vi "UHR-Fleezers Control (fpga) - Leonardo 04-2018 V5.2.vi"() -> ()   [LabVIEW 2013]
doc: "UHR-Fleezers Instrument Control Code (fpga)"
uses:
  <vilib>/Platform/TimedLoop/XDataNode/timing_clust.ctl
  <vilib>/Platform/TimedLoop/XDataNode/nitl_modes.ctl
  <vilib>/Platform/TimedLoop/XDataNode/wakeup.ctl
  <vilib>/rvi/eio/common/nirviEmuTemplateMethod_errors.vi
  <vilib>/rvi/Emulation/niFpgaSctlEmulationGetInTimedLoop.vi
  <vilib>/rvi/Emulation/niFpgaEmulationReportErrorSimple.vi
  <vilib>/rvi/Emulation/niFpgaGetClockAttributes.vi
  <vilib>/rvi/Emulation/niFpgaCriticalErrorInLSC.vi
  <vilib>/rvi/FIFO/Fifo_Resource/nirvififoEmulationReadFpgaImpl.vi
  <vilib>/rvi/DataTransferAndStorage/Container/Common/niFpgaContainerGetUniqueNameForEmu.vi
  <vilib>/rvi/DataTransferAndStorage/Container/Common/niFpgaContainerExecOnDevCompGetState.vi
  <vilib>/rvi/interface/RandomDataEmulation/nirviRandomDataFPGAFIFO.vi
  <vilib>/rvi/interface/RandomDataEmulation/niFpgaRandomDataHandleErrors.vi
  <vilib>/rvi/eio/common/nirviEmuReportErrorAndStop.vi
  <vilib>/rvi/Emulation/niFpgaProcessEmulError.vi
  <vilib>/rvi/FIFO/Fifo_Resource/nirvififoEmulationWriteFpgaImpl.vi
  <vilib>/Platform/TimedLoop/XDataNode/XDataNode.xnode
  <vilib>/eio/EIOMethodNode/EIOMethodNode.xnode
  <vilib>/eio/EIONode/EIONode.xnode
  <vilib>/rvi/DataTransferAndStorage/Container/XNode/niFpgaContainer.xnode
  <vilib>/rvi/FIFO/Fifo_Resource/nirvififoEmulationRead.vi
  <vilib>/rvi/FIFO/Fifo_Resource/niFpgaFifoEmulationRefIn.vi
  <vilib>/rvi/interface/RandomDataEmulation/nirviRandomDataFpgaReadWriteTemplate.vi
  <vilib>/rvi/FIFO/Fifo_Resource/nirvififoEmulationWrite.vi
  <vilib>/addons/control/pid/fpga.llb/XNode/niFpgaPID.xnode
  <vilib>/Platform/TimedLoop/XDataNode/XDNodeRunTimeDep.lvlib
  <vilib>/rvi/Memory/Memory_Emulation/niFpgaMemoryEmulationRefIn.vi
panel:
  in  "Symmetric FB/Raster":bool
  in  "Tab Control 2":T1(tab)
  out "BD1 amplitude 1 out":u16
  out "BD1 amplitude 2 out":u16
  in  "FB output range":cluster{"output low":i16, "output high":i16}={"output low"=0, "output high"=3000}
  in  "FB Gains":T2={"proportional gain (Kc)"=10, "integral gain (Kc*Ts/Ti)"=5, "derivative gain (Kc*Td/Ts)"=0}
  in  "RF synth green feedback max":i16=4000
  in  "RD":bool=TRUE
  in  "Swap F1 and F2":bool
  in  "Scan BD":bool
  in  "Start scan":bool
  in  "OSK Bd 1":bool
  in  "Reset Bd 1":bool
  in  "PMODE":bool=TRUE
  in  "Number Interlace Cycles":u8=2 min=1 max=3
  in  "Interlace Off Parameters":u8=1 min=1 max=3
  in  "Interlace ON/OFF":bool
  out "DIO Relative phase":i16
  in  "Phase count adjustment (DIO)":i16
  in  "+ phase (DIO)":bool
  out "DIO Late Counter":u8
  in  "DIO count 1 (ticks)":u16=400
  in  "DIO count 2 (ticks)":u16=400
  in  "DIO count 3 (ticks)":u16=400
  out "AI2 Y Sum Set 2":i16
  out "AI2 Y Sum Set 1":i16
  in  "FB Setpoint Set 1":i16 min=0 step=1
  in  "FB Reset Set 1":bool
  in  "FB On/Off Set 1":bool
  in  "FB Reset Set 2":bool
  in  "FB On/Off Set 2":bool
  in  "FB Setpoint Set 2":i16 min=0 step=1
  in  "Amp switch delay":u8=5
  in  "RF synth bd controls green":bool
  in  "Phase Trap 2":fxp<+,14,14>
  in  "Phase Trap 1":fxp<+,14,14>
  in  "Phase offset method":u8
  in  "BD 2 Amplitude 1":u16
  in  "BD 1 Amplitude 1":u16
  in  "BD 2 Frequency 1":u64
  in  "BD 1 Frequency 1":u64
  in  "BD 2 Amplitude 2":u16
  in  "BD 1 Amplitude 2":u16
  in  "BD 2 Frequency 2":u64
  in  "BD 1 Frequency 2":u64
  in  "BD 2 Amplitude 3":u16
  in  "BD 1 Amplitude 3":u16
  in  "BD 2 Frequency 3":u64
  in  "BD 1 Frequency 3":u64
  in  "BD 2 Delay (Ticks)":u8 caption="Count(Ticks)"
  in  "Next trap write delay (ticks)":u8 caption="Count(Ticks)"
  out "Random phase generated":fxp<+,14,14>
  in  "RF phase reset before cycles":bool
  in  "Trap 1 osc enable":bool
  in  "N trap osc periods":i16
  in  "Trap osc period (pts)":i16
  in  "Osc traps":bool
  in  "Initiate trap osc":bool
  in  "Ready Write":bool
  in  "Data":i64
  in  "Address 2":u32
  in  "Osc trap cont.":bool
  in  "Trap 2 osc enable":bool
  out "green FB running":bool
  in  "APD 2 AO scale factor":i16=1
  in  "BD 1 Delay (ticks)":u8
  in  "Tab Control":T3(tab)=enum."MCL trap control"
  in  "Set 3":bool
  in  "Set 2":bool=TRUE
  in  "Set 1":bool=TRUE
  in  "Trap Pos to FIFO":bool
  in  "N of AI1 Int Acq Sets":i16=2 min=1 max=3 step=1
  out "AI Late Counter":u8
  in  "ai count":u16=400
  in  "+ phase":bool
  in  "Phase count adjustment":i16
  out "Relative phase":i16
  in  "AI to FIFO":bool
  out "BD1 Frequency Out 1":u64
  out "BD1 Frequency Out 2":u64
  out "Trap Pos FIFO Timeout":u16
  out "Trap AI FIFO Timeout":u16
  in  "Trap FIFO Set Timeout":i32
  in  "Scan freq.  increment":i64
  in  "Scan steps":u64
  in  "Number of scans":u16
  in  "Cycles per step":u64
  in  "Raster setpoint":fxp<+/-,16,1>
  in  "Raster to target force":bool
  out "Actual Scan freq":u64
  in  "Cont. Scan":bool
  out "Scan I":u64
  in  "Abort scan":bool
  out "Scanning":bool
  in  "FB Min frequency":u64
  in  "FB Max Frequency":u64
  in  "Dynamic Force FB (Ronen)":bool
  in  "Trap pos. FB Range":T4={"FB2 output low"=-1.0, "FB2 output high"=0.999969482421875}
  in  "Trap Pos. FB Gains":T5={"proportional gain (Kc)"=0.999969482421875, "integral gain (Kc*Ts/Ti)"=0.999969482421875, "derivative gain (Kc*Td/Ts)"=0.0}
  in  "B factor":fxp<+/-,32,16>
  in  "Negate Diff?":bool
  in  "Diff FB Measurement?":bool
  in  "FB Trig Integrate":u32=1
  out "TTrig?":bool
  in  "TTrig Negate Pos":bool=TRUE
  out "Trap Pos FB Int Signal":fxp<+/-,24,9> format="%.18g"
  out "Trap Pos FB Int-Norm Signal":fxp<+/-,16,1> format="%.16g"
  in  "FPGA TTrig Thresh":i64
  in  "FPGA Trap Trig":bool
  out "Trap Pos FB Action":i64
  in  "Trap Pos. FB Offset Factor":i64
  in  "Trap Pos. FB Mult Factor":i64=2
  in  "Trap Pos. FB Reset":bool
  in  "Trap Pos FB Monitor T1 or T2":bool
  in  "AI1 X Scale":u16
  in  "Trap Pos FB Int Count":u16=100
  in  "Trap Pos FB Negate Action":bool
  out "AI1 X Set 2":fxp<+/-,16,1>
  out "AI1 X Set 1":fxp<+/-,16,1>
  in  "Trap Pos. FB SP":fxp<+/-,16,1>
  in  "Force feedback":bool
  out "TTrig Sig":i64
  out "TTrig Fin Thresh":i64
  in  "1D or 2D Scan?":bool
  in  "Abort scan (MCL)":bool
  in  "MCL Scan Axis":bool
  in  "Cont. Scan (MCL)":bool
  out "Scan I (MCL)":u64
  in  "Number of scans (MCL)":u16
  out "Scanning MCL":bool
  in  "Scan steps (MCL)":u64
  in  "Cycles per step (MCL)":u64
  in  "Scan freq.  increment (MCL)":i16
  in  "Start scan (MCL)":bool
  in  "AO2 (X)":i16
  in  "AO1 (Y)":i16
  out "MCL Late Counter":u8
  in  "MCL count":u32=800
  out "MCL Relative Phase":i16
  in  "Phase count adjustment (MCL)":i16
  in  "+ phase (MCL)":bool
  in  "Lifetime events to read blue":u16=100
  in  "Lifetime read blue fifo":bool
  out "lifetime events in fifo":u16
  out "APD2 int gate":bool
  in  "APD Gate Operating Mode":u8 max=2 step=1
  in  "Invert APD Gate":bool
  in  "APD Gate OFF Count":u16=100
  in  "APD Gate ON Count":u16=300
  out "APD 1 Gate Late Counter":u8
  out "APD 1 Gate Relative Phase":i16
  in  "Phase count adjustment (APD 1 Gate)":i16
  in  "+ phase (APD 1 Gate)":bool
  out "APD 2 Counts 0":u32
  out "APD 2 Counts 1":u32
  out "APD 1 Counts 0":u32
  out "APD 1 Counts 1":u32
  in  "Phase count adjustment (APD 2 Gate)":i16
  out "APD 2 Gate Late Counter":u8
  out "APD 2 Gate Relative Phase":i16
  in  "+ phase (APD 2 Gate)":bool
  out "APD 3 Counts 0":u32
  out "APD 3 Counts 1":u32
  out "APD 3 Gate Late Counter":u8
  in  "Phase count adjustment (APD 3 Gate)":i16
  out "APD 3 Gate Relative Phase":i16
  in  "+ phase (APD 3 Gate)":bool
  out "APD1 int gate":bool
  out "APD3 int gate":bool
  in  "Lifetime timeout APD1":u16=200
  in  "APD to FIFO":bool
  in  "APD Acq Rate Count":u32=20000000
  out "APD Acq Late Counter":u16
  out "APD Acq Relative Phase":i16
  in  "+ phase (APD Acq)":bool
  in  "Phase Count Adjustment (APD Acq)":i16
  in  "APD 1 AO scale factor":i16=1
  out "APD2 out state":bool
  out "APD1 out state":bool
  out "APD Acq Late?":bool
  in  "Number of OFF cycles":i16
  in  "Green long-scale interlacing":bool
  in  "D3 2":i16
  in  "I3 2":i16=5
  in  "P3 2":i16=10
  in  "Green FB Setpoint 2":i16=250 min=0 step=1
  in  "Green FB Reset 2":bool
  in  "Green Filter Flipper":bool
  in  "Green interlace OFF count":u16=100
  out "GI Relative phase":i16
  in  "Phase count adjustment (GI)":i16
  in  "+ phase (GI)":bool
  in  "Green interlace ON count":u16=300
  out "GI Late Counter":u8
  in  "Invert GI":bool
  in  "Operating Mode":u8 max=2 step=1
  in  "Current Out":u16=30000
  in  "Green int current ON count adj":u32=150
  in  "Green interlace OFF count 2":u32=900
  in  "Green interlace ON count 2":u32=300
  out "GI Late Counter 2":u16
  in  "Green FB Count":u32=1200
  in  "Phase count adjustment (GI) 2":i16=20
  in  "Green FB Setpoint":i16=250 min=0 step=1
  in  "Invert GI 2":bool
  out "GI Relative phase 2":i16
  in  "+ phase (GI) 2":bool
  in  "Phase count adjustment (Green FB)":i16=10
  out "Green Late Counter":u16
  out "Green FB Relative Phase":i16
  in  "+ phase (Green FB)":bool
  out "Green FB Signals":T6
  out "Green FB Sum":i16
  in  "Green FB Gains":T2={"proportional gain (Kc)"=10, "integral gain (Kc*Ts/Ti)"=5, "derivative gain (Kc*Td/Ts)"=0}
  in  "Green FB On/Off":bool
  in  "Green FB Reset":bool
  out "Green FB Late?":bool
  out "GI Late?":bool
  in  "Operating Mode 2":u8=2 max=2 step=1
  in  "Chassis2/Mod4/AO1":u16
  in  "Number of ON cycles":i16
  in  "+ phase (RI)":bool
  out "RI Relative phase":i16
  out "RI Late Counter":u8
  in  "Red interlace ON count":u16=300
  in  "Red interlace OFF count":u16=100
  in  "Invert RI":bool
  in  "Red Laser Operating Mode":u8 max=2 step=1
  in  "Phase count adjustment (RI)":i16
  in  "Phase count adjustment (BI D)":i16
  in  "Blue Laser Operating Mode (D)":u8 max=2 step=1
  in  "Invert BI (D)":bool
  in  "Blue interlace OFF count (D)":u16=100
  in  "Blue interlace ON count (D)":u16=300
  out "Blue Late Counter (D)":u8
  out "BI Relative phase (D)":i16
  in  "+ phase (BI D)":bool
  in  "Lifetime to FIFO":bool
  out "lifetime (ticks)":u16
  # "Raster Scan AOD"
  # "1 (X)"
  # "2 (Y)"
  # "IR Intensity Feedback (RF BD 1)"
  # "FB Gains Set 1"
  # "FB output range 1"
  # "IR Intensity Feedback (RF BD 2) -\nonly when using BD 2 for green laser AOM (not trap Y)"
  # "Keep below 4096 (12 bits) to stay within range of RF board. Going over doesn't saturate, it truncates higher bits."
  # "RF phase offset control"
  # "Methods are:\n0 - Default, do nothing at all (no phase offset writes)\n1 - Manual phase adjustment\n2 - Cycle the phase adjustment using the input phase numbers as increment values for each cycle"
  # "False is usual, True is external loop method"
  # "Parameters if using the external RF switching loop"
  # "Parameters if using the usual internal RF switching method"
  # "FB Triggering Excitation Laser"
  # "Trap Pos. FB Gains"
  # "Trap Pos. FB Range"
  # "AO1 (Y)"
  # "2D"
  # "Trap 3"
  # "1D"
  # "AO2 (X)"
  # "Fl Laser"
  # "APD AO for aligning"
  # "Detection Loop"
  # "Green fluorescent laser digital gate interlacing loop"
  # "0 Forced ON\n1 Forced OFF\n2 Interlacing"
  # "ALEX settings:"
  # "Controls for usual IA ME controls green AOM"
  # "Controls for RF synth board controls green AOM"
  # "Green FB Gains"
  # "Red fluorescent laser digital gate interlacing loop"
  # "Detection Loop"
  # "0 Forced ON\n1 Forced OFF\n2 Interlacing"
  # "Analog/FB Control Loop\n(Disabled)"
  # "Digital Control Loop"
  # "Blue laser intensity reading"
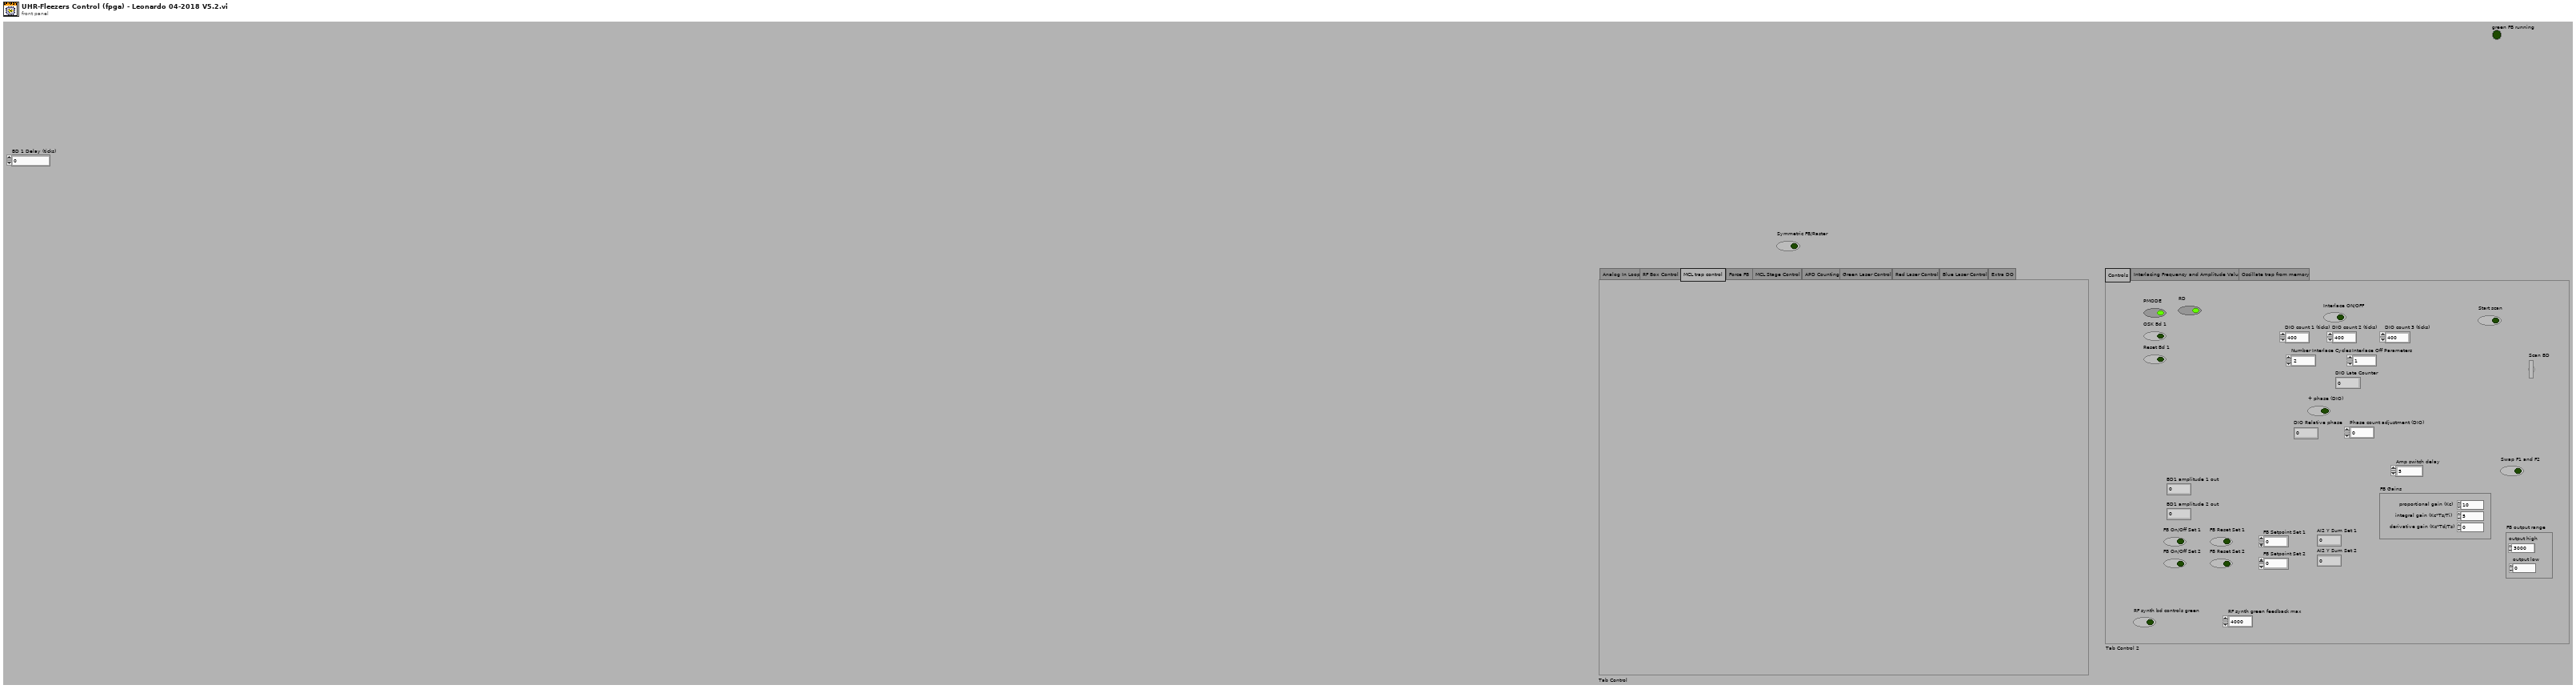
[diagram p1: front panel]
types:
  T1 = enum32{"Controls", "Interlacing Frequency and Amplitude Values", "Oscillate trap from memory"}
  T2 = cluster{"proportional gain (Kc)":i16, "integral gain (Kc*Ts/Ti)":i16, "derivative gain (Kc*Td/Ts)":i16}
  T3 = enum32{"Analog In Loop", "RF Box Control", "MCL trap control", "Force FB", "MCL Stage Control", "APD Counting", "Green Laser Control", "Red Laser Control", "Blue Laser Control", "Extra DO"}
  T4 = cluster{"FB2 output low":fxp<+/-,16,1>, "FB2 output high":fxp<+/-,16,1>}
  T5 = cluster{"proportional gain (Kc)":fxp<+/-,16,1>, "integral gain (Kc*Ts/Ti)":fxp<+/-,16,1>, "derivative gain (Kc*Td/Ts)":fxp<+/-,16,1>}
  T6 = cluster{"Green FB Ch 0":i16, "Green FB Ch 1":i16, "Green FB Ch 2":i16}
  T7 = typedef "XDNodeRunTimeDep.lvlib/timing_clust.ctl" = cluster{"Expected End [f-1]":u64, "Actual End [f-1]":u64, "Finished Late? [f-1]":bool, "Expected End [i-1]":u64, "Actual End [i-1]":u64, "Finished Late? [i-1]":bool, "Expected Start [i]":u64, "Actual Start [i]":u64, "Expected Start [f]":u64, "Actual Start [f]":u64, "Source Name":string, "Structure Name":string, "Period":i64, "Deadline":i64, "Offset":i64, "Start":i64, "Priority":i32, "Timeout":i32, "Mode":T8, "Wakeup Reason":T9, "Error":errorcluster, "Source Type":string, "Secondary Source Type":string, "Global End Time":u64, "Global Start Time":u64, "Frame Duration":u64, "Iteration Duration":u64, "Assigned CPU":i32, "I/O Scan Engine Mode":u32}
  T8 = typedef "XDNodeRunTimeDep.lvlib/nitl_modes.ctl" = enum32{"No Change", "Process missed periods, maintain original phase", "Discard missed periods, maintain original phase", "Process missed periods, ignore original phase", "Discard missed periods, ignore original phase"}
  T9 = typedef "XDNodeRunTimeDep.lvlib/wakeup.ctl" = enum32{"Normal", "Aborted", "Asynchronous wakeup", "Timing source error", "Timed loop error", "Timeout"}
  T10 = cluster{"Chassis2/Mod2/AI0":i16, "Chassis2/Mod2/AI1":i16, "Chassis2/Mod2/AI2":i16}
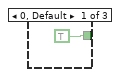
[diagram p2: hidden frame]
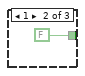
[diagram p3: hidden frame]
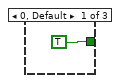
[diagram p6: hidden frame]
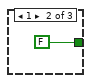
[diagram p7: hidden frame]
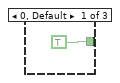
[diagram p11: hidden frame]
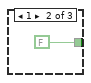
[diagram p12: hidden frame]
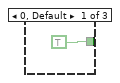
[diagram p13: hidden frame]
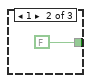
[diagram p14: hidden frame]
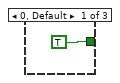
[diagram p18: hidden frame]
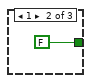
[diagram p19: hidden frame]
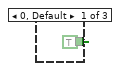
[diagram p20: hidden frame]
diagram:
  w4 = FALSE
  w5 = FALSE
  # "BD2 amp"
  # "BD1 amp"
  # "BD2 amp"
  # "BD1 amp"
  # "timing array current index"
  # "timing array"
  # "timing counter (phase adjusted here)"
  # "late counter"
  n1 = while {
    stop <- FALSE stop-if-true
    n2 = xnode "FPGA I/O Node"("Connector0/DIO3"="Green Filter Flipper", "Chassis2/Mod1/AO1"="Chassis2/Mod4/AO1") -> ()  [unwired: 2 in, 2 out]
    n3 = call "Loop Timer11"("Count(Ticks)"=u32 40000 ("Extra DO Counts")) -> ()  [unwired: 1 out]
  }
  n4 = disable-structure shown="Disabled" {
    frame Disabled {
      w19 = i16 2 items=["UnSet Ready", "ReadWrite", "Wait Ready"]
      n5 = while "Handshake memory transfer for trap oscillation sin wave data" {
        shift-right: [w21] -> _
        shift-left: w19 -> [w22]
        stop <- FALSE stop-if-true
        # "Write"
        n6 = case shown="1" w22 {
          tunnel: [w25 w30 w31] -> w21
          frame 3, Default {
            w23 = i16 2 items=["UnSet Ready", "ReadWrite", "Wait Ready"]
            w24 = i16 1 items=["UnSet Ready", "ReadWrite", "Wait Ready"]
            n7 = Select(t=w24, s="Ready Write", f=w23) -> (s? t:f=w25:i16)
          }
          frame 1 {
            w30 = i16 0 items=["UnSet Ready", "ReadWrite", "Wait Ready"]
            n8 = xnode ("Memory Write")("Address"="Address 2", "Data"="Data", "Memory In"=refnum<k21> "Trap osc memory") -> ()  [unwired: 1 out]
          }
          frame 0 {
            w31 = i16 2 items=["UnSet Ready", "ReadWrite", "Wait Ready"]
            n9 = local write "Ready Write"(FALSE ("Ready Read")) -> ()
          }
        }
      }
    }
    frame Enabled {
    }
  }
  n10 = flat-sequence "FPGA initialization to do before running any of the loops" {
    tunnel: [u16 0 ("DIO count 3 (ticks)")] -> w3
    tunnel: [w40] -> _
    frame #0 {
      # "UDCLK out enable and set low"
      # "WR"
      # "BD 2"
      # "BD 1"
      # "With the RF synth board initialization now done in a separate fpga vi, now when this vi is started, board is already configured and is ready for interlacing. Just need to set WR high and enabled UDCLK as write and set to low.\nbefore setting data and address bits."
      # "Start up expansion chassis early\nto avoid delays later"
      # "Set data and address values to something safe (a correct setting) so any initial WR and udclk flipping doesn't have a chance to mess anything up. Safe would be setting an unused data entry:"
      n11 = xnode "FPGA I/O Method Node"("Enable"=TRUE) -> ("FPGA I/O Out"=w34:refnum<k21>)  [unwired: 1 in]
      n12 = xnode "FPGA I/O Method Node"("Enable"=TRUE) -> ("FPGA I/O Out"=w37:refnum<k21>)  [unwired: 1 in]
      n13 = xnode "FPGA I/O Node"("Chassis2/Mod1/AO0"=u16 0 ("Chassis2/Mod4/AO0")) -> ("Chassis2/Mod2/AI0"=w40:i16)  [unwired: 2 in, 2 out]
      n14 = xnode "FPGA I/O Node"("Connector1/DIO15"=TRUE) -> ()  [unwired: 1 in, 1 out]
      n15 = xnode "FPGA I/O Node"("I/O Item"=FALSE ("Connector1/DIO30"), "FPGA I/O In"=w34) -> ()  [unwired: 1 out]
      n16 = xnode "FPGA I/O Node"("I/O Item"=FALSE ("Connector1/DIO30"), "FPGA I/O In"=w37) -> ()  [unwired: 1 out]
      n17 = xnode "FPGA I/O Node"("Connector1/DIO0"=FALSE, "Connector1/DIO1"=FALSE, "Connector1/DIO2"=FALSE, "Connector1/DIO3"=FALSE, "Connector1/DIO4"=FALSE, "Connector1/DIO5"=FALSE, "Connector1/DIO6"=FALSE, "Connector1/DIO7"=FALSE, "Connector1/DIO8"=FALSE, "Connector1/DIO9"=FALSE, "Connector1/DIO10"=FALSE, "Connector1/DIO11"=FALSE, "Connector1/DIO12"=FALSE, "Connector1/DIO13"=FALSE, "Connector1/DIO20"=FALSE, "Connector1/DIO21"=FALSE, "Connector1/DIO22"=FALSE, "Connector1/DIO23"=FALSE, "Connector1/DIO24"=FALSE, "Connector1/DIO25"=FALSE, "Connector1/DIO26"=FALSE, "Connector1/DIO27"=FALSE, "Connector1/DIO14"=FALSE) -> ()  [unwired: 23 in, 23 out]
    }
  }
  n18 = node-c288() -> (w11:T7)  [unwired: 1 in]
  n19 = timed-loop "RF box board DIO control: control bits" {
    timing: w11 -> [_]
    timing-out: [_] -> w10
    tunnel: [w67] -> _
    tunnel: w3 -> [w67]
    stop <- FALSE stop-if-true
    n20 = xnode "FPGA I/O Node"("Connector1/DIO16"="RD", "Connector1/DIO17"="PMODE", "Connector1/DIO18"="OSK Bd 1", "Connector1/DIO19"="Reset Bd 1") -> ()  [unwired: 4 in, 4 out]
  }
  n21 = node-c288(w10) -> ()
  n22 = local read "AO1 (Y)"() -> (w13:i16)
  n23 = local read "AO2 (X)"() -> (w12:i16)
  n24 = To Unsigned Long Integer(number=w3) -> (unsigned 32bit integer=w6:u32)
  n25 = disable-structure shown="Disabled" {
    disable-tunnel: w5 -> [w75 _]
    disable-tunnel: w3 -> [w74 _]
    frame Disabled {
      n26 = while "APD 2 Gating" {
        shift-right: [w79] -> _
        shift-left: w74 -> [w84]
        shift-right: [w78] -> _
        shift-left: w75 -> [w76]
        stop <- FALSE stop-if-true
        n27 = flat-sequence {
          tunnel: w84 -> [w87]
          tunnel: [w88] -> w82
          tunnel: [w87] -> w80
          tunnel: [w86] -> w77
          tunnel: w76 -> [w86]
          tunnel: [w91] -> w83
          tunnel: w82 -> [w91]
          tunnel: [w90] -> w81
          tunnel: w80 -> [w90]
          tunnel: w77 -> [w89]
          tunnel: [w113] -> w79
          tunnel: w83 -> [w123]
          tunnel: w81 -> [w121]
          tunnel: [w92] -> w78
          frame #0 {
            n28 = call "Loop Timer3"("Count(Ticks)"=w87) -> ("Tick Count(Ticks)"=w88:u32)
          }
          frame #1 {
            # "Signal maybe then sent through \na transistor before APD"
            n29 = xnode "FPGA I/O Node"("Connector1/DIO34"=w89) -> ()  [unwired: 1 in, 1 out]
            "APD2 int gate" <- w89
          }
          frame #2 {
            n30 = local read "APD Gate ON Count"() -> (w106:u16)
            n31 = local read "APD Gate OFF Count"() -> (w105:u16)
            n32 = feedback #1(TRUE) -> (w118:bool)
            n33 = feedback-in #2(w123) -> ()
            n34 = feedback #2(w123) -> (w107:u32)
            n35 = Not(x=w118) -> (.not. x?=w116:bool)
            n36 = feedback-in #1(w116) -> ()
            n37 = Subtract(x=w123, y=w107) -> (x-y=w122:u32)
            n38 = Select(t=w106, s=w116, f=w105) -> (s? t:f=w120:u16)
            n39 = Subtract(x=w122, y=w121) -> (x-y=w98:u32)
            n40 = Subtract(x=w120, y=w98) -> (x-y=w112:u32)
            n41 = Number To Boolean Array(number=w98) -> (Boolean array=w97:bool[])
            n42 = Or Array Elements(Boolean array=w97) -> (logical OR=w96:bool)
            n43 = Boolean To (0,1)(Boolean="+ phase (APD 2 Gate)") -> (0, 1=w110:i16)
            n44 = Multiply(x=w110, y="Phase count adjustment (APD 2 Gate)") -> (x*y=w108:i16)
            n45 = Boolean To (0,1)(Boolean=w96) -> (0, 1=w103:i16)
            n46 = Add(x=w112, y=w108) -> (x+y=w113:u32)
            n47 = To Unsigned Byte Integer(number=w103) -> (unsigned 8bit integer=w100:u8)
            n48 = feedback #3(i16 0) -> (w115:i16)
            n49 = Subtract(x=w115, y=w108) -> (x-y=w114:i16)
            "APD 2 Gate Relative Phase" <- w114
            n50 = feedback-in #3(w114) -> ()
            n51 = feedback #4(u8 0) -> (w101:u8)
            n52 = Add(x=w100, y=w101) -> (x+y=w99:u8)
            "APD 2 Gate Late Counter" <- w99
            n53 = feedback-in #4(w99) -> ()
            n54 = local read "APD Gate Operating Mode"() -> (w104:u8)
            n55 = case shown="2" w104 {
              tunnel: [TRUE FALSE w126] -> w93
              tunnel: w118 -> [_ _ w126]
              frame 0, Default {
              }
              frame 1 {
              }
              frame 2 {
              }
            }
            n56 = local read "Invert APD Gate"() -> (w95:bool)
            n57 = Not(x=w93) -> (.not. x?=w94:bool)
            n58 = Select(t=w94, s=w95, f=w93) -> (s? t:f=w92:bool)
          }
        }
      }
    }
    frame Enabled {
    }
  }
  n59 = while "DAQ AI set 1" {
    shift-right: [w127] -> _
    shift-left: w3 -> [w132]
    stop <- FALSE stop-if-true
    n60 = flat-sequence {
      tunnel: w132 -> [w143]
      tunnel: [w142] -> w130
      tunnel: [w143] -> w129
      tunnel: [w153] -> w140
      tunnel: [w152] -> w139
      tunnel: [w151] -> w138
      tunnel: [w150] -> w137
      tunnel: [w149] -> w136
      tunnel: [w148] -> w135
      tunnel: [w147] -> w134
      tunnel: [w146] -> w133
      tunnel: [w145] -> w131
      tunnel: w130 -> [w145]
      tunnel: w129 -> [w144]
      tunnel: [w144] -> w128
      tunnel: [w183] -> w127
      tunnel: w140 -> [w209]
      tunnel: w139 -> [w175]
      tunnel: w138 -> [w176]
      tunnel: w137 -> [w155]
      tunnel: w136 -> [w199]
      tunnel: w135 -> [w198]
      tunnel: w134 -> [w197]
      tunnel: w133 -> [w196]
      tunnel: w131 -> [w193]
      tunnel: w128 -> [w190]
      frame #0 {
        n61 = call "Loop Timer"("Count(Ticks)"=w143) -> ("Tick Count(Ticks)"=w142:u32)
      }
      frame #1 {
        n62 = xnode "FPGA I/O Node"("Connector1/DIO31"=TRUE ("Connector1/DIO33")) -> ("Connector0/AI0"=w153:i16, "Connector0/AI1"=w152:i16, "Connector0/AI2"=w151:i16, "Connector0/AI3"=w150:i16, "Connector0/AI4"=w149:i16, "Connector0/AI5"=w148:i16, "Connector0/AI6"=w147:i16, "Connector0/AI7"=w146:i16)  [unwired: 9 in, 9 out]
      }
      frame #2 {
        w179 = FALSE ("AI to FIFO")
        # "Normalize by trap bead QPD sum, AI3"
        # "Adjust phase after data acquired if button pressed"
        n63 = feedback #5(i16 1) -> (w202:i16)
        n64 = Increment(x=w202) -> (x+1=w208:i16)
        n65 = Scale By Power Of 2(n="AI1 X Scale", x=w175) -> (x*2^n=w173:i16)
        n66 = Greater?(x=w208, y="N of AI1 Int Acq Sets") -> (0:w205:bool)
        n67 = Select(t=i16 1, s=w205, f=w208) -> (s? t:f=w207:i16)
        n68 = feedback-in #5(w207) -> ()
        n69 = Divide(x=w173, y=w155) -> (x/y=w172:fxp<+/-,16,1>)
        n70 = feedback #6(w179) -> (w177:bool)
        n71 = feedback #7(w179) -> (w195:bool)
        n72 = case shown="1, Default" w202 {
          tunnel: w176 -> [w232 w239 _]
          tunnel: ["Set 1" "Set 2" "Set 3"] -> w200
          tunnel: ["AI to FIFO" w241 w246] -> w194
          tunnel: w195 -> [_ w241 w246]
          tunnel: ["Trap Pos to FIFO" w240 w245] -> w178
          tunnel: w177 -> [_ w240 w245]
          tunnel: w172 -> [w231 w238 _]
          tunnel: [w230 w236 FALSE] -> w159
          tunnel: [w229 w237 u64 0 ("BD1 Frequency Out 2")] -> w158
          frame 1, Default {
            n73 = local read "BD1 Frequency Out 1"() -> (w229:u64)
            n74 = Compound Arithmetic op=AND("Trap Pos to FIFO", "Set 1", "AI to FIFO") -> (w230:bool)
            "AI2 Y Sum Set 1" <- w232
            "AI1 X Set 1" <- w231
          }
          frame 2 {
            n75 = local read "BD1 Frequency Out 2"() -> (w237:u64)
            n76 = Compound Arithmetic op=AND(w240, "Set 2", w241) -> (w236:bool)
            "AI2 Y Sum Set 2" <- w239
            "AI1 X Set 2" <- w238
          }
          frame 3 {
          }
        }
        n77 = And(x=w200, y=w194) -> (x .and. y?=w201:bool)
        n78 = case shown="True" w201 {
          tunnel: w209 -> [_ w260]
          tunnel: w175 -> [_ w259]
          tunnel: w176 -> [_ w258]
          tunnel: w155 -> [_ w257]
          tunnel: w199 -> [_ w256]
          tunnel: w198 -> [_ w255]
          tunnel: w197 -> [_ w254]
          tunnel: w196 -> [_ w253]
          tunnel: 0 ("DMA buffer timeout") -> [_ w262]
          frame False {
          }
          frame True {
            n79 = Build Array(w260, w259, w258, w257, w256, w255, w254, w253) -> (w261:i16[])
            n80 = for {
              tunnel: w261 -> [w264] mode=indexing
              tunnel: w262 -> [w265]
              tunnel: [w263] -> w251 mode=indexing
              n81 = xnode ("FIFO Write")("Element"=w264, "Timeout"=w265) -> ("Timed Out?"=w263:bool)  [unwired: 1 in, 1 out]
            }
            n82 = Or Array Elements(Boolean array=w251) -> (logical OR=w248:bool)
            n83 = Boolean To (0,1)(Boolean=w248) -> (0, 1=w250:i16)
            n84 = feedback #8(u16 0) -> (w249:u16)
            n85 = Add(x=w250, y=w249) -> (x+y=w247:u16)
            "Trap AI FIFO Timeout" <- w247
            n86 = feedback-in #8(w247) -> ()
          }
        }
        n87 = feedback-in #6(w178) -> ()
        n88 = feedback-in #7(w194) -> ()
        n89 = case shown="True" w159 {
          tunnel: w158 -> [_ w215]
          tunnel: [u8 0 w212] -> w157
          frame False {
          }
          frame True {
            n90 = Split Number(x=w215) -> (hi(x)=w216:u32, lo(x)=w217:u32)
            n91 = Split Number(x=w216) -> (lo(x)=w218:u16)  [unwired: 1 out]
            n92 = Split Number(x=w217) -> (hi(x)=w219:u16, lo(x)=w220:u16)
            n93 = Build Array "BD 1 nu Stack"(w218, w219, w220) -> (w214:u16[])
            n94 = for {
              tunnel: w214 -> [w227] mode=indexing
              shift-right: [w223] -> w212
              shift-left: u8 0 -> [w224]
              n95 = xnode ("FIFO Method Node")("Element"=w227, "Timeout"="Trap FIFO Set Timeout") -> ("Timed Out?"=w226:bool)  [unwired: 1 in, 1 out]
              n96 = Boolean To (0,1)(Boolean=w226) -> (0, 1=w225:i16)
              n97 = To Unsigned Byte Integer(number=w225) -> (unsigned 8bit integer=w222:u8)
              n98 = Add(x=w222, y=w224) -> (x+y=w223:u8)
            }
          }
        }
        n99 = To Unsigned Word Integer(number=w157) -> (unsigned 16bit integer=w156:u16)
        n100 = feedback #9(u16 0) -> (w170:u16)
        n101 = Add(x=w156, y=w170) -> (x+y=w169:u16)
        "Trap Pos FIFO Timeout" <- w169
        n102 = feedback-in #9(w169) -> ()
        n103 = feedback-in #10(w193) -> ()
        n104 = feedback #10(w193) -> (w192:u32)
        n105 = Subtract(x=w193, y=w192) -> (x-y=w191:u32)
        n106 = xnode "FPGA I/O Node"("Connector1/DIO31"=FALSE ("Connector1/DIO34")) -> ()  [unwired: 1 in, 1 out]
        n107 = Subtract(x=w191, y=w190) -> (x-y=w161:u32)
        n108 = Boolean To (0,1)(Boolean="+ phase") -> (0, 1=w186:i16)
        n109 = Multiply(x=w186, y="Phase count adjustment") -> (x*y=w180:i16)
        n110 = Subtract(x="ai count", y=w161) -> (x-y=w184:u32)
        n111 = Number To Boolean Array(number=w161) -> (Boolean array=w162:bool[])
        n112 = feedback #11(i16 0) -> (w182:i16)
        n113 = Add(x=w184, y=w180) -> (x+y=w183:u32)
        n114 = Subtract(x=w182, y=w180) -> (x-y=w181:i16)
        "Relative phase" <- w181
        n115 = feedback-in #11(w181) -> ()
        n116 = Or Array Elements(Boolean array=w162) -> (logical OR=w160:bool)
        n117 = Boolean To (0,1)(Boolean=w160) -> (0, 1=w167:i16)
        n118 = To Unsigned Byte Integer(number=w167) -> (unsigned 8bit integer=w164:u8)
        n119 = feedback #12(u8 0) -> (w165:u8)
        n120 = Add(x=w164, y=w165) -> (x+y=w163:u8)
        "AI Late Counter" <- w163
        n121 = feedback-in #12(w163) -> ()
      }
    }
  }
  n122 = while "MCL stage control" {
    shift-right: [w278] -> _
    shift-left: w3 -> [w281]
    shift-right: [w271] -> _
    shift-left: w13 -> [w268]
    shift-right: [w270] -> _
    shift-left: w12 -> [w266]
    stop <- FALSE stop-if-true
    n123 = flat-sequence {
      tunnel: w281 -> [w284]
      tunnel: [w283] -> w277
      tunnel: [w284] -> w275
      tunnel: [w286] -> w269
      tunnel: w268 -> [w286]
      tunnel: [w285] -> w267
      tunnel: w266 -> [w285]
      tunnel: w277 -> [w290]
      tunnel: [w290] -> w276
      tunnel: w275 -> [w289]
      tunnel: [w289] -> w274
      tunnel: w269 -> [w288]
      tunnel: w267 -> [w287]
      tunnel: w276 -> [w298]
      tunnel: w274 -> [w297]
      tunnel: [w298] -> w280
      tunnel: [w297] -> w279
      tunnel: [w296] -> w273
      tunnel: [w295] -> w272
      tunnel: [w370] -> w278
      tunnel: w280 -> [w377]
      tunnel: w279 -> [w374]
      tunnel: w273 -> [w372]
      tunnel: w272 -> [w371]
      tunnel: [w372] -> w271
      tunnel: [w371] -> w270
      frame #0 {
        n124 = call "Loop Timer3"("Count(Ticks)"=w284) -> ("Tick Count(Ticks)"=w283:u32)
      }
      frame #1 {
        n125 = xnode "FPGA I/O Node"("Connector0/AO1"=w288, "Connector0/AO2"=w287) -> ()  [unwired: 2 in, 2 out]
      }
      frame #2 {
        n126 = local read "Scanning MCL"() -> (w310:bool)
        n127 = Or(x=w310, y="Start scan (MCL)") -> (x .or. y?=w305:bool)
        n128 = Not(x="Abort scan (MCL)") -> (.not. x?=w303:bool)
        n129 = And(x=w303, y=w305) -> (x .and. y?=w302:bool)
        n130 = case "Raster scan" shown="False" w302 {
          tunnel: [w311 w354] -> w307
          tunnel: "Start scan (MCL)" -> [_ w339]
          tunnel: [w311 w315] -> w291
          frame False {
            w311 = i16 0
            n131 = local write "Scanning MCL"(FALSE ("scanning")) -> ()
          }
          frame True {
            w325 = i16 0
            w324 = u64 0
            # "scan incr."
            # "freq. incr. mult."
            # "count steps"
            # "count number of cycles"
            n132 = feedback #13(w324) -> (w351:u64)
            n133 = Select(t=w324, s=w339, f=w351) -> (s? t:f=w353:u64)
            n134 = Increment(x=w353) -> (x+1=w350:u64)
            n135 = Greater?(x="Cycles per step (MCL)", y=w350) -> (0:w334:bool)
            n136 = Select(t=w350, s=w334, f=w324) -> (s? t:f=w349:u64)
            n137 = feedback-in #13(w349) -> ()
            n138 = feedback #14(w324) -> (w348:u64)
            n139 = Select(t=w324, s=w339, f=w348) -> (s? t:f=w343:u64)
            n140 = Increment(x=w343) -> (x+1=w347:u64)
            n141 = Add(x="Scan steps (MCL)", y="Scan steps (MCL)") -> (x+y=w346:u64)
            n142 = Select(t=w343, s=w334, f=w347) -> (s? t:f=w329:u64)
            n143 = Greater?(x=w346, y=w329) -> (0:w328:bool)
            n144 = Select(t=w329, s=w328, f=w324) -> (s? t:f=w344:u64)
            n145 = feedback-in #14(w344) -> ()
            n146 = Equal?(x="Scan steps (MCL)", y=w329) -> (x = y?=w333:bool)
            n147 = Greater?(x="Scan steps (MCL)", y=w343) -> (0:w342:bool)
            n148 = feedback #15(w325) -> (w345:i16)
            n149 = Select(t=w325, s=w339, f=w345) -> (s? t:f=w331:i16)
            n150 = Increment(x=w331) -> (x+1=w341:i16)
            n151 = Decrement(x=w331) -> (x-1=w340:i16)
            n152 = Select(t=w341, s=w342, f=w340) -> (s? t:f=w332:i16)
            n153 = Select(t=w331, s=w333, f=w332) -> (s? t:f=w330:i16)
            n154 = Select(t=w331, s=w334, f=w330) -> (s? t:f=w326:i16)
            n155 = Select(t=w326, s=w328, f=w325) -> (s? t:f=w327:i16)
            n156 = feedback-in #15(w327) -> ()
            n157 = feedback #16(w324) -> (w338:u64)
            n158 = Select(t=w324, s=w339, f=w338) -> (s? t:f=w313:u64)
            n159 = Increment(x=w313) -> (x+1=w335:u64)
            n160 = Select(t=w313, s=w328, f=w335) -> (s? t:f=w314:u64)
            n161 = Greater?(x="Number of scans (MCL)", y=w314) -> (0:w321:bool)
            n162 = Multiply(x="Scan freq.  increment (MCL)", y=w331) -> (x*y=w354:i16)
            n163 = Select(t=TRUE, s="Cont. Scan (MCL)", f=w321) -> (s? t:f=w320:bool)
            "Scanning MCL" <- w320
            n164 = Select(t=w314, s=w320, f=w324) -> (s? t:f=w336:u64)
            n165 = feedback-in #16(w336) -> ()
            n166 = Increment(x=w314) -> (x+1=→"Scan I (MCL)":u64)
            n167 = To Word Integer(number=w313) -> (16bit integer=w316:i16)
            n168 = Multiply(x=w316, y="Scan freq.  increment (MCL)") -> (x*y=w315:i16)
          }
        }
        n169 = Select(t=w291, s="1D or 2D Scan?", f=i16 0) -> (s? t:f=w292:i16)
        n170 = Select(t=w307, s="MCL Scan Axis", f=w292) -> (s? t:f=w308:i16)
        n171 = Select(t=w292, s="MCL Scan Axis", f=w307) -> (s? t:f=w306:i16)
        n172 = Add(x="AO2 (X)", y=w306) -> (x+y=w295:i16)
        n173 = Add(x="AO1 (Y)", y=w308) -> (x+y=w296:i16)
      }
      frame #3 {
        n174 = feedback-in #17(w377) -> ()
        n175 = feedback #17(w377) -> (w376:u32)
        n176 = Boolean To (0,1)(Boolean="+ phase (MCL)") -> (0, 1=w368:i16)
        n177 = Subtract(x=w377, y=w376) -> (x-y=w375:u32)
        n178 = Multiply(x=w368, y="Phase count adjustment (MCL)") -> (x*y=w364:i16)
        n179 = Subtract(x=w375, y=w374) -> (x-y=w356:u32)
        n180 = Subtract(x="MCL count", y=w356) -> (x-y=w366:u32)
        n181 = feedback #18(i16 0) -> (w365:i16)
        n182 = Subtract(x=w365, y=w364) -> (x-y=w363:i16)
        "MCL Relative Phase" <- w363
        n183 = feedback-in #18(w363) -> ()
        n184 = Number To Boolean Array(number=w356) -> (Boolean array=w357:bool[])
        n185 = Or Array Elements(Boolean array=w357) -> (logical OR=w355:bool)
        n186 = Boolean To (0,1)(Boolean=w355) -> (0, 1=w362:i16)
        n187 = Add(x=w366, y=w364) -> (x+y=w370:u32)
        n188 = To Unsigned Byte Integer(number=w362) -> (unsigned 8bit integer=w359:u8)
        n189 = feedback #19(u8 0) -> (w360:u8)
        n190 = Add(x=w359, y=w360) -> (x+y=w358:u8)
        "MCL Late Counter" <- w358
        n191 = feedback-in #19(w358) -> ()
      }
    }
  }
  n192 = while "APD 2 Counter" {
    tunnel: w3 -> [_]
    stop <- FALSE stop-if-true
    n193 = flat-sequence {
      frame #0 {
        n194 = xnode "FPGA I/O Method Node"("FPGA I/O In"=refnum<k21> "Connector0/DIO1" ("APD 2 DO"), "Timeout"=-1) -> ()  [unwired: 2 out]
      }
      frame #1 {
        n195 = local read "APD1 int gate"() -> (w382:bool)
        n196 = case shown="True" w382 {
          frame False {
          }
          frame True {
            n197 = local read "APD2 out state"() -> (w383:bool)
            n198 = case shown="True" w383 {
              frame False {
                n199 = local read "APD 2 Counts 0"() -> (w385:u32)
                n200 = Increment(x=w385) -> (x+1=→"APD 2 Counts 0":u32)
              }
              frame True {
                n201 = local read "APD 2 Counts 1"() -> (w387:u32)
                n202 = Increment(x=w387) -> (x+1=→"APD 2 Counts 1":u32)
              }
            }
          }
        }
      }
    }
  }
  n203 = while "Green fluorescent laser interlacing (Current to IA 532 nm AOM ME amp)." {
    shift-right: [w393] -> _
    shift-left: w3 -> [w396]
    shift-right: [w390] -> _
    shift-left: i16 0 -> [w388]
    stop <- FALSE stop-if-true
    n204 = flat-sequence {
      tunnel: w396 -> [w399]
      tunnel: [w400] -> w395
      tunnel: [w399] -> w394
      tunnel: [w398] -> w389
      tunnel: w388 -> [w398]
      tunnel: [w403] -> w392
      tunnel: w395 -> [w403]
      tunnel: [w402] -> w391
      tunnel: w394 -> [w402]
      tunnel: w389 -> [w401]
      tunnel: [w416] -> w393
      tunnel: [w432] -> w390
      tunnel: w392 -> [w445]
      tunnel: w391 -> [w442]
      frame #0 {
        n205 = call "Loop Timer10"("Count(Ticks)"=w399) -> ("Tick Count(Ticks)"=w400:u32)
      }
      frame #1 {
        n206 = xnode "FPGA I/O Node"("Chassis2/Mod1/AO0"=w401) -> ()  [unwired: 1 in, 1 out]
      }
      frame #2 {
        n207 = local read "RF synth bd controls green"() -> (w407:bool)
        n208 = Subtract(x="Green interlace OFF count 2", y="Green int current ON count adj") -> (x-y=w425:u32)
        n209 = feedback-in #20(w445) -> ()
        n210 = feedback #20(w445) -> (w444:u32)
        n211 = Add(x="Green int current ON count adj", y="Green interlace ON count 2") -> (x+y=w426:u32)
        n212 = Subtract(x=w445, y=w444) -> (x-y=w443:u32)
        n213 = Subtract(x=w443, y=w442) -> (x-y=w409:u32)
        n214 = Not(x=w407) -> (.not. x?=w405:bool)
        n215 = Number To Boolean Array(number=w409) -> (Boolean array=w410:bool[])
        n216 = Boolean To (0,1)(Boolean="+ phase (GI) 2") -> (0, 1=w422:i16)
        n217 = Or Array Elements(Boolean array=w410) -> (logical OR=w408:bool)
        "GI Late?" <- w408
        n218 = Boolean To (0,1)(Boolean=w408) -> (0, 1=w415:i16)
        n219 = Multiply(x=w422, y="Phase count adjustment (GI) 2") -> (x*y=w418:i16)
        n220 = To Unsigned Word Integer(number=w415) -> (unsigned 16bit integer=w411:u16)
        n221 = feedback #21(u16 0) -> (w413:u16)
        n222 = Add(x=w411, y=w413) -> (x+y=w412:u16)
        "GI Late Counter 2" <- w412
        n223 = feedback-in #21(w412) -> ()
        n224 = feedback #22(i16 0) -> (w419:i16)
        n225 = Subtract(x=w419, y=w418) -> (x-y=w417:i16)
        "GI Relative phase 2" <- w417
        n226 = feedback-in #22(w417) -> ()
        n227 = feedback #23(TRUE) -> (w437:bool)
        n228 = case shown="2" "Operating Mode 2" {
          tunnel: [TRUE FALSE w462] -> w427
          tunnel: w437 -> [_ _ w459]
          frame 0, Default {
          }
          frame 1 {
          }
          frame 2 {
            n229 = Not(x=w459) -> (.not. x?=w461:bool)
            n230 = Select(t=w461, s="Invert GI 2", f=w459) -> (s? t:f=w462:bool)
          }
        }
        n231 = And(x=w427, y="Green FB On/Off") -> (x .and. y?=w406:bool)
        "green FB running" <- w406
        n232 = And(x=w406, y=w405) -> (x .and. y?=w404:bool)
        n233 = case shown="True" w404 {
          tunnel: "Current Out" -> [w446 _]
          tunnel: [w446 w451] -> w431
          frame False {
          }
          frame True {
            n234 = local read "Green FB Sum"() -> (w447:i16)
            n235 = call "Slower PID.vi"("process variable"=w447, "reset?"="Green FB Reset", "setpoint"="Green FB Setpoint", "PID gains (x 2^8)"="Green FB Gains", "output range"=cluster{"output high":i16, "output low":i16} {"output high"=32767, "output low"=-32768} ("Green FB output range")) -> ("output"=w455:i16)  [unwired: 10 out]
            n236 = To Long Integer(number=w455) -> (32bit integer=w448:i32)
            n237 = Add(x=w448, y=32768) -> (x+y=w450:i32)
            n238 = To Unsigned Word Integer(number=w450) -> (unsigned 16bit integer=w451:u16)
          }
        }
        n239 = Not(x=w437) -> (.not. x?=w434:bool)
        n240 = Select(t=w426, s=w434, f=w425) -> (s? t:f=w439:u32)
        n241 = Subtract(x=w439, y=w409) -> (x-y=w420:u32)
        n242 = Add(x=w420, y=w418) -> (x+y=w416:u32)
        n243 = feedback-in #23(w434) -> ()
        n244 = Boolean To (0,1)(Boolean=w427) -> (0, 1=w433:i16)
        n245 = To Unsigned Word Integer(number=w433) -> (unsigned 16bit integer=w430:u16)
        n246 = Multiply(x=w430, y=w431) -> (x*y=w432:u16)
      }
    }
  }
  n247 = while "APD 1 Counter" {
    tunnel: w3 -> [_]
    stop <- FALSE stop-if-true
    n248 = flat-sequence {
      frame #0 {
        n249 = xnode "FPGA I/O Method Node"("FPGA I/O In"=refnum<k21> "Connector0/DIO0" ("APD 1 DO"), "Timeout"=-1) -> ()  [unwired: 2 out]
      }
      frame #1 {
        n250 = local read "APD1 int gate"() -> (w466:bool)
        n251 = case shown="True" w466 {
          frame False {
          }
          frame True {
            n252 = local read "APD1 out state"() -> (w467:bool)
            n253 = case shown="True" w467 {
              frame False {
                n254 = local read "APD 1 Counts 0"() -> (w469:u32)
                n255 = Increment(x=w469) -> (x+1=→"APD 1 Counts 0":u32)
              }
              frame True {
                n256 = local read "APD 1 Counts 1"() -> (w471:u32)
                n257 = Increment(x=w471) -> (x+1=→"APD 1 Counts 1":u32)
              }
            }
          }
        }
      }
    }
  }
  n258 = while "RF synth board interlacing timing loop" {
    tunnel: w3 -> [_]
    stop <- FALSE stop-if-true
    # "This loop is stalled until the RF FIFO get a value. With this method we gain additional delay time (because  we allow the rest of the main RF loop to procede while this loop waits to send the switch signals - a form of parallelism). This helps to simplify the main RF code. \n\nThe code also allow optimal interlacing while also controlling trap RF phase. \n\nNote: a lot of work has gone into optimizing these methods and it is unclear how they can be made any faster or better than this (many failed tries). Right now there is essentially ~4 ticks (~90 ns ns) of imperfection in the switching from trap 1 to trap 2. ~2 ticks of no RF (phase reset) then ~2 ticks of trap 2 with the wrong amplitude (T1 amplitude). The total ticks is 200, so not a big error.\n\nPhase can be precisely set for each trap. Phase reset and switching, has similar delays as fsk frequency switching. And phase reset and phase offset changes are also not simultaneous. So we can't perfectly line everything up.\n\nIf you start from amp zero though (as for trap 1), the on switch is perfect. Likewise the off is perfect for trap 2. \n\nThe green laser switching is also perfect because of its reduced duty cycle and delays in fsk switching between 80 and 0 MHz."
    n259 = xnode ("FIFO Read")("Timeout"=-1) -> ("Element"=w518:u16, "FIFO Out"=w514:refnum<k21>)  [unwired: 1 in, 1 out]
    n260 = Equal To 0?(x=w518) -> (x = 0?=w515:bool)
    n261 = Not(x=w515) -> (.not. x?=w472:bool)
    n262 = flat-sequence "BD 1 and 2 RF phase and amplitude switching" {
      tunnel: w472 -> [_]
      tunnel: w507 -> [w622]
      tunnel: w506 -> [w621]
      tunnel: w505 -> [w620]
      tunnel: w504 -> [w619]
      tunnel: w503 -> [w618]
      tunnel: w502 -> [w617]
      tunnel: w501 -> [w616]
      tunnel: w500 -> [w615]
      tunnel: w498 -> [w614]
      tunnel: w497 -> [w613]
      tunnel: w496 -> [w612]
      tunnel: w494 -> [w610]
      tunnel: w493 -> [w609]
      tunnel: w492 -> [w608]
      tunnel: w495 -> [w611]
      tunnel: w499 -> [w607]
      tunnel: w491 -> [w646]
      tunnel: w490 -> [w645]
      tunnel: w489 -> [w644]
      tunnel: w488 -> [w643]
      tunnel: w487 -> [w642]
      tunnel: w486 -> [w641]
      tunnel: w485 -> [w640]
      tunnel: w484 -> [w639]
      tunnel: w483 -> [w638]
      tunnel: w481 -> [w637]
      tunnel: w480 -> [w636]
      tunnel: w479 -> [w635]
      tunnel: w478 -> [w634]
      tunnel: w477 -> [w633]
      tunnel: w476 -> [w632]
      tunnel: w482 -> [w631]
      frame #0 {
        # "Delay to align amp/frequency switching depending on the method used.\n\nCan also give enough time to do the parallel amplitude calculations"
        n263 = call "Wait2"("Count(Ticks)"="Amp switch delay") -> ()  [unwired: 1 out]
      }
      frame #1 {
        w602 = TRUE ("Connector1/DIO30")
        # "make phase offset and phase reset active with buffer transfer"
        n264 = xnode "FPGA I/O Node"("Connector1/DIO29"=w602, "Connector1/DIO30"=w602) -> ()  [unwired: 2 in, 2 out]
      }
      frame #2 {
        w603 = FALSE ("Connector1/DIO15")
        # "write phase restart to buffer and reset udclk"
        n265 = xnode "FPGA I/O Node"("Connector1/DIO29"=w603, "Connector1/DIO30"=w603, "Connector1/DIO15"=FALSE ("Connector1/DIO14")) -> ()  [unwired: 3 in, 3 out]
      }
      frame #3 {
        w605 = TRUE ("Connector1/DIO15")
        # "make phase restart active"
        # "reset WR"
        n266 = xnode "FPGA I/O Node"("Connector1/DIO15"=w605, "Connector1/DIO29"=w605, "Connector1/DIO30"=w605) -> ()  [unwired: 3 in, 3 out]
      }
      frame #4 {
        w606 = FALSE ("Connector1/DIO30")
        # "Address"
        # "set amp byte 1, and reset udclk"
        n267 = xnode "FPGA I/O Node"("Connector1/DIO0"=w622, "Connector1/DIO1"=w621, "Connector1/DIO2"=w620, "Connector1/DIO3"=w619, "Connector1/DIO4"=w618, "Connector1/DIO5"=w617, "Connector1/DIO6"=w616, "Connector1/DIO7"=w615, "Connector1/DIO8"=TRUE, "Connector1/DIO9"=FALSE, "Connector1/DIO10"=FALSE, "Connector1/DIO11"=FALSE, "Connector1/DIO12"=FALSE, "Connector1/DIO13"=TRUE, "Connector1/DIO20"=w607, "Connector1/DIO21"=w614, "Connector1/DIO22"=w613, "Connector1/DIO23"=w612, "Connector1/DIO24"=w611, "Connector1/DIO25"=w610, "Connector1/DIO26"=w609, "Connector1/DIO27"=w608, "Connector1/DIO30"=w606, "Connector1/DIO29"=w606) -> ()  [unwired: 24 in, 24 out]
      }
      frame #5 {
        # "write amp byte 1 to buffer"
        n268 = xnode "FPGA I/O Node"("Connector1/DIO15"=FALSE ("Connector1/DIO14")) -> ()  [unwired: 1 in, 1 out]
      }
      frame #6 {
        # "reset WR"
        n269 = xnode "FPGA I/O Node"("Connector1/DIO15"=TRUE) -> ()  [unwired: 1 in, 1 out]
      }
      frame #7 {
        # "Address"
        # "set amp byte 2"
        n270 = xnode "FPGA I/O Node"("Connector1/DIO0"=w646, "Connector1/DIO1"=w645, "Connector1/DIO2"=w644, "Connector1/DIO3"=w643, "Connector1/DIO4"=w642, "Connector1/DIO5"=w641, "Connector1/DIO6"=w640, "Connector1/DIO7"=w639, "Connector1/DIO8"=TRUE, "Connector1/DIO9"=FALSE, "Connector1/DIO10"=FALSE, "Connector1/DIO11"=FALSE, "Connector1/DIO12"=TRUE, "Connector1/DIO13"=FALSE, "Connector1/DIO20"=w638, "Connector1/DIO21"=w631, "Connector1/DIO22"=w637, "Connector1/DIO23"=w636, "Connector1/DIO24"=w635, "Connector1/DIO25"=w634, "Connector1/DIO26"=w633, "Connector1/DIO27"=w632) -> ()  [unwired: 22 in, 22 out]
      }
      frame #8 {
        # "write amp byte 2"
        n271 = xnode "FPGA I/O Node"("Connector1/DIO15"=FALSE ("Connector1/DIO14")) -> ()  [unwired: 1 in, 1 out]
      }
      frame #9 {
        w654 = TRUE ("Connector1/DIO15")
        # "transfer amp bytes 1 and 2 and reset WR"
        n272 = xnode "FPGA I/O Node"("Connector1/DIO29"=w654, "Connector1/DIO30"=w654, "Connector1/DIO15"=TRUE ("Connector1/DIO14")) -> ()  [unwired: 3 in, 3 out]
      }
      frame #10 {
        w656 = FALSE ("Connector1/DIO14")
        # "reset udclk"
        n273 = xnode "FPGA I/O Node"("Connector1/DIO29"=w656, "Connector1/DIO30"=w656) -> ()  [unwired: 2 in, 2 out]
      }
    }
    n274 = flat-sequence "FSK BD 1 (trap X)" {
      tunnel: w472 -> [w520]
      tunnel: [w520] -> w475
      tunnel: w475 -> [w521]
      frame #0 {
        n275 = call "Wait"("Count(Ticks)"="BD 1 Delay (ticks)") -> ()  [unwired: 1 out]
      }
      frame #1 {
        # "switch frequency"
        n276 = xnode "FPGA I/O Node"("Connector1/DIO36"=w521) -> ()  [unwired: 1 in, 1 out]
      }
    }
    n277 = flat-sequence "FSK BD 2 (trap Y or green laser AOM)" {
      tunnel: w472 -> [w658]
      tunnel: [w658] -> w517
      tunnel: w517 -> [w659]
      frame #0 {
        n278 = call "Wait3"("Count(Ticks)"="BD 2 Delay (Ticks)") -> ()  [unwired: 1 out]
      }
      frame #1 {
        # "switch frequency"
        n279 = xnode "FPGA I/O Node"("Connector1/DIO37"=w659) -> ()  [unwired: 1 in, 1 out]
      }
    }
    n280 = xnode ("FIFO Read")("Timeout"=-1, "FIFO In"=w514) -> ("Element"=w509:u16, "FIFO Out"=w513:refnum<k21>)  [unwired: 1 out]
    n281 = xnode ("FIFO Read")("Timeout"=-1, "FIFO In"=w513) -> ("Element"=w508:u16)  [unwired: 2 out]
    n282 = node-c288() -> (w511:T7)  [unwired: 1 in]
    n283 = timed-loop "Convert amplitude words to bits" {
      timing: w511 -> [_]
      timing-out: [_] -> w510
      tunnel: w509 -> [w578]
      tunnel: w508 -> [w577]
      tunnel: [w554] -> w507
      tunnel: [w553] -> w506
      tunnel: [w552] -> w505
      tunnel: [w551] -> w504
      tunnel: [w550] -> w503
      tunnel: [w549] -> w502
      tunnel: [w548] -> w501
      tunnel: [w547] -> w500
      tunnel: [w546] -> w499
      tunnel: [w545] -> w498
      tunnel: [w544] -> w497
      tunnel: [w543] -> w496
      tunnel: [w542] -> w495
      tunnel: [w541] -> w494
      tunnel: [w540] -> w493
      tunnel: [w539] -> w492
      tunnel: [w538] -> w491
      tunnel: [w537] -> w490
      tunnel: [w536] -> w489
      tunnel: [w535] -> w488
      tunnel: [w534] -> w487
      tunnel: [w533] -> w486
      tunnel: [w532] -> w485
      tunnel: [w531] -> w484
      tunnel: [w530] -> w483
      tunnel: [w529] -> w482
      tunnel: [w528] -> w481
      tunnel: [w527] -> w480
      tunnel: [w526] -> w479
      tunnel: [w525] -> w478
      tunnel: [w524] -> w477
      tunnel: [w523] -> w476
      stop <- TRUE stop-if-true
      # "Board 1 Data"
      # "Board 2 Data"
      # "Board 1 Data"
      # "Board 2 Data"
      n284 = Split Number(x=w578) -> (hi(x)=w576:u8, lo(x)=w556:u8)
      n285 = Split Number(x=w577) -> (hi(x)=w575:u8, lo(x)=w555:u8)
      n286 = Number To Boolean Array(number=w576) -> (Boolean array=w596:bool[])
      n287 = Number To Boolean Array(number=w575) -> (Boolean array=w587:bool[])
      n288 = Index Array(array=w596, index=7) -> (element=w554:bool)
      n289 = Index Array(array=w596, index=6) -> (element=w553:bool)
      n290 = Index Array(array=w596, index=5) -> (element=w552:bool)
      n291 = Index Array(array=w596, index=4) -> (element=w551:bool)
      n292 = Index Array(array=w596, index=3) -> (element=w550:bool)
      n293 = Index Array(array=w596, index=2) -> (element=w549:bool)
      n294 = Index Array(array=w596, index=1) -> (element=w548:bool)
      n295 = Index Array(array=w596, index=0) -> (element=w547:bool)
      n296 = Index Array(array=w587, index=7) -> (element=w546:bool)
      n297 = Index Array(array=w587, index=6) -> (element=w545:bool)
      n298 = Index Array(array=w587, index=5) -> (element=w544:bool)
      n299 = Index Array(array=w587, index=4) -> (element=w543:bool)
      n300 = Index Array(array=w587, index=3) -> (element=w542:bool)
      n301 = Index Array(array=w587, index=2) -> (element=w541:bool)
      n302 = Index Array(array=w587, index=1) -> (element=w540:bool)
      n303 = Index Array(array=w587, index=0) -> (element=w539:bool)
      n304 = Number To Boolean Array(number=w556) -> (Boolean array=w574:bool[])
      n305 = Number To Boolean Array(number=w555) -> (Boolean array=w565:bool[])
      n306 = Index Array(array=w574, index=7) -> (element=w538:bool)
      n307 = Index Array(array=w574, index=6) -> (element=w537:bool)
      n308 = Index Array(array=w574, index=5) -> (element=w536:bool)
      n309 = Index Array(array=w574, index=4) -> (element=w535:bool)
      n310 = Index Array(array=w574, index=3) -> (element=w534:bool)
      n311 = Index Array(array=w574, index=2) -> (element=w533:bool)
      n312 = Index Array(array=w574, index=1) -> (element=w532:bool)
      n313 = Index Array(array=w574, index=0) -> (element=w531:bool)
      n314 = Index Array(array=w565, index=7) -> (element=w530:bool)
      n315 = Index Array(array=w565, index=6) -> (element=w529:bool)
      n316 = Index Array(array=w565, index=5) -> (element=w528:bool)
      n317 = Index Array(array=w565, index=4) -> (element=w527:bool)
      n318 = Index Array(array=w565, index=3) -> (element=w526:bool)
      n319 = Index Array(array=w565, index=2) -> (element=w525:bool)
      n320 = Index Array(array=w565, index=1) -> (element=w524:bool)
      n321 = Index Array(array=w565, index=0) -> (element=w523:bool)
    }
    n322 = node-c288(w510) -> ()
  }
  n323 = while "APD 1 Gating" {
    shift-right: [w663] -> _
    shift-left: w3 -> [w668]
    shift-right: [w662] -> _
    shift-left: w5 -> [w660]
    stop <- FALSE stop-if-true
    n324 = flat-sequence {
      tunnel: w668 -> [w671]
      tunnel: [w672] -> w666
      tunnel: [w671] -> w664
      tunnel: [w670] -> w661
      tunnel: w660 -> [w670]
      tunnel: [w675] -> w667
      tunnel: w666 -> [w675]
      tunnel: [w674] -> w665
      tunnel: w664 -> [w674]
      tunnel: w661 -> [w673]
      tunnel: [w695] -> w663
      tunnel: w667 -> [w709]
      tunnel: w665 -> [w706]
      tunnel: [w677] -> w662
      frame #0 {
        n325 = call "Loop Timer4"("Count(Ticks)"=w671) -> ("Tick Count(Ticks)"=w672:u32)
      }
      frame #1 {
        # "Signal maybe then sent through \na transistor before APD"
        n326 = xnode "FPGA I/O Node"("Connector1/DIO33"=w673) -> ()  [unwired: 1 in, 1 out]
        "APD1 int gate" <- w673
      }
      frame #2 {
        n327 = feedback #24(TRUE) -> (w701:bool)
        n328 = feedback-in #25(w709) -> ()
        n329 = feedback #25(w709) -> (w708:u32)
        n330 = Not(x=w701) -> (.not. x?=w698:bool)
        n331 = feedback-in #24(w698) -> ()
        n332 = Subtract(x=w709, y=w708) -> (x-y=w707:u32)
        n333 = Select(t="APD Gate ON Count", s=w698, f="APD Gate OFF Count") -> (s? t:f=w703:u16)
        n334 = Subtract(x=w707, y=w706) -> (x-y=w683:u32)
        n335 = Subtract(x=w703, y=w683) -> (x-y=w694:u32)
        n336 = Number To Boolean Array(number=w683) -> (Boolean array=w684:bool[])
        n337 = Or Array Elements(Boolean array=w684) -> (logical OR=w682:bool)
        n338 = Boolean To (0,1)(Boolean="+ phase (APD 1 Gate)") -> (0, 1=w692:i16)
        n339 = Boolean To (0,1)(Boolean=w682) -> (0, 1=w689:i16)
        n340 = Multiply(x=w692, y="Phase count adjustment (APD 1 Gate)") -> (x*y=w690:i16)
        n341 = To Unsigned Byte Integer(number=w689) -> (unsigned 8bit integer=w686:u8)
        n342 = Add(x=w694, y=w690) -> (x+y=w695:u32)
        n343 = feedback #26(i16 0) -> (w697:i16)
        n344 = Subtract(x=w697, y=w690) -> (x-y=w696:i16)
        "APD 1 Gate Relative Phase" <- w696
        n345 = feedback-in #26(w696) -> ()
        n346 = feedback #27(u8 0) -> (w687:u8)
        n347 = Add(x=w686, y=w687) -> (x+y=w685:u8)
        "APD 1 Gate Late Counter" <- w685
        n348 = feedback-in #27(w685) -> ()
        n349 = local read "Green long-scale interlacing"() -> (w676:bool)
        n350 = case shown="2" "APD Gate Operating Mode" {
          tunnel: [TRUE FALSE w731] -> w679
          tunnel: w701 -> [_ _ w731]
          frame 0, Default {
          }
          frame 1 {
          }
          frame 2 {
          }
        }
        n351 = Not(x=w679) -> (.not. x?=w680:bool)
        n352 = Select(t=w680, s="Invert APD Gate", f=w679) -> (s? t:f=w678:bool)
        n353 = case shown="True" w676 {
          tunnel: w678 -> [w710 w718]
          tunnel: [w710 w719] -> w677
          frame False {
          }
          frame True {
            n354 = local read "Number of ON cycles"() -> (w712:i16)
            n355 = local read "Number of OFF cycles"() -> (w714:i16)
            n356 = feedback #28(i16 1) -> (w725:i16)
            n357 = Increment(x=w725) -> (x+1=w724:i16)
            n358 = feedback #29(w712) -> (w711:i16)
            n359 = Greater?(x=w711, y=w725) -> (0:w720:bool)
            n360 = Select(t=w724, s=w720, f=i16 1) -> (s? t:f=w722:i16)
            n361 = feedback-in #28(w722) -> ()
            n362 = feedback #30(TRUE) -> (w717:bool)
            n363 = Not(x=w717) -> (.not. x?=w716:bool)
            n364 = Select(t=w717, s=w720, f=w716) -> (s? t:f=w715:bool)
            n365 = feedback-in #30(w715) -> ()
            n366 = Select(t=w712, s=w715, f=w714) -> (s? t:f=w713:i16)
            n367 = feedback-in #29(w713) -> ()
            n368 = case shown="True" w715 {
              tunnel: [FALSE w728] -> w719
              tunnel: w718 -> [_ w728]
              frame False {
              }
              frame True {
              }
            }
          }
        }
      }
    }
  }
  n369 = while "Trap RF control, main calculations (raster scanning, intensity and position feedback, phase control etc) with primary timing trigger" {
    shift-right: [w748] -> _
    shift-left: w3 -> [w747]
    shift-right: [w746] -> _
    shift-left: FALSE ("Swap F1 and F2") -> [w745]
    shift-right: [w741] -> _
    shift-left: u16 0 ("BD 1 Amplitude 3") -> [w738]
    shift-right: [w740] -> _
    shift-left: u16 0 ("BD 2 Amplitude 3") -> [w736]
    shift-right: [w735] -> _
    shift-left: u64 0 -> [w734]
    shift-right: [w733] -> _
    shift-left: u64 0 -> [w732]
    stop <- FALSE stop-if-true
    n370 = flat-sequence {
      tunnel: w745 -> [w754]
      tunnel: w747 -> [w751]
      tunnel: [w754] -> w744
      tunnel: [w750] -> w743
      tunnel: [w751] -> w742
      tunnel: [w753] -> w739
      tunnel: w738 -> [w753]
      tunnel: [w752] -> w737
      tunnel: w736 -> [w752]
      tunnel: [w767] -> w748
      tunnel: [w766] -> w746
      tunnel: w744 -> [w765]
      tunnel: w743 -> [w764]
      tunnel: w742 -> [w763]
      tunnel: [w762] -> w741
      tunnel: [w761] -> w740
      tunnel: w739 -> [w760]
      tunnel: w737 -> [w759]
      tunnel: [w758] -> w735
      tunnel: w734 -> [w757]
      tunnel: [w756] -> w733
      tunnel: w732 -> [w755]
      frame #0 {
        n371 = call "Loop Timer2"("Count(Ticks)"=w751) -> ("Tick Count(Ticks)"=w750:u32)
      }
      frame #1 {
        n372 = flat-sequence {
          tunnel: w765 -> [w775]
          tunnel: w760 -> [w769]
          tunnel: w759 -> [w768]
          tunnel: [w837] -> w767
          tunnel: [w849] -> w766
          tunnel: w764 -> [w843]
          tunnel: w763 -> [w840]
          tunnel: [w788] -> w762
          tunnel: [w787] -> w761
          tunnel: [w779] -> w758
          tunnel: w757 -> [w778]
          tunnel: [w777] -> w756
          tunnel: w755 -> [w776]
          frame #0 {
            w770 = -1 ("Timeout")
            # "Operation when you need a long delay for either X or Y to synchonize AOD light out phase (> ~100 ticks)\nor want shorter trap ON timing. Puts some of the delay timing in parallel with the later computations."
            # "Trigger the external loop by sending the boolean FSK value through a FIFO.\nTiming is precise."
            n373 = Boolean To (0,1)(Boolean=w775) -> (0, 1=w774:i16)
            n374 = To Unsigned Word Integer(number=w774) -> (unsigned 16bit integer=w773:u16)
            n375 = xnode ("FIFO Method Node")("Element"=w773, "Timeout"=w770) -> ("FIFO Out"=w772:refnum<k21>)  [unwired: 1 in, 1 out]
            n376 = xnode ("FIFO Method Node")("Element"=w769, "Timeout"=w770, "FIFO In"=w772) -> ("FIFO Out"=w771:refnum<k21>)  [unwired: 1 out]
            n377 = xnode ("FIFO Method Node")("Element"=w768, "Timeout"=w770, "FIFO In"=w771) -> ()  [unwired: 2 out]
          }
          frame #1 {
            # "Just counts, wraps around, 8 bit"
            # "Which trap cycle"
            # "Only save the 3rd set's amp in the loop"
            # "If this is NOT set 3 AND NOT (RF synth controls green AND green FB running)\nthen use this sets amp value (otherwise keep the green feedback value)"
            # "Just flips back and forth."
            # "If interlacing is off, this is which cycle to use."
            # "Keep track of trap cycles (trap 1, 2, 3...)"
            # "This is the prior cycle's on time"
            # "increment timing\nindex, reset to 0 if \nend of matrix"
            # "Reset to begginning (1) when number of cycles reached."
            # "timing index"
            # "build byte stacks for writing data\n(must correspond to addresses array constant)"
            # "Timing housekeeping"
            # "Adjust phase if late\n(maintains constant phase relationship between cycles)"
            n378 = feedback #31(u8 0 ("t")) -> (w846:u8)
            n379 = Increment(x=w846) -> (x+1=w885:u8)
            n380 = Increment(x="Number Interlace Cycles") -> (x+1=w880:u8)
            n381 = Equal?(x=w885, y=w880) -> (x = y?=w887:bool)
            n382 = Select(t=u8 1, s=w887, f=w885) -> (s? t:f=w845:u8)
            n383 = feedback-in #31(w845) -> ()
            n384 = Increment(x=w845) -> (x+1=w882:u8)
            n385 = Equal?(x=w882, y=w880) -> (x = y?=w883:bool)
            n386 = Select "This cycle"(t=u8 1, s=w883, f=w882) -> (s? t:f=w879:u8)
            n387 = Select(t=w879, s="Interlace ON/OFF", f="Interlace Off Parameters") -> (s? t:f=w798:u8)
            n388 = feedback-in #32(w843) -> ()
            n389 = feedback #32(w843) -> (w842:u32)
            n390 = Select(t=w845, s="Interlace ON/OFF", f="Interlace Off Parameters") -> (s? t:f=w878:u8)
            n391 = Subtract(x=w843, y=w842) -> (x-y=w841:u32)
            n392 = Subtract "The error"(x=w841, y=w840) -> (x-y=w824:u32)
            n393 = case shown="1, Default" w878 {
              tunnel: ["DIO count 1 (ticks)" "DIO count 2 (ticks)" "DIO count 3 (ticks)"] -> w839
              frame 1, Default {
              }
              frame 2 {
              }
              frame 3 {
              }
            }
            n394 = Number To Boolean Array(number=w824) -> (Boolean array=w825:bool[])
            n395 = Or Array Elements(Boolean array=w825) -> (logical OR=w823:bool)
            n396 = Boolean To (0,1)(Boolean=w823) -> (0, 1=w830:i16)
            n397 = To Unsigned Byte Integer(number=w830) -> (unsigned 8bit integer=w827:u8)
            n398 = feedback #33(u8 0) -> (w828:u8)
            n399 = Add(x=w827, y=w828) -> (x+y=w826:u8)
            "DIO Late Counter" <- w826
            n400 = feedback-in #33(w826) -> ()
            n401 = Subtract(x=w839, y=w824) -> (x-y=w838:u32)
            n402 = disable-structure shown="Disabled" {
              disable-tunnel: [w891 _] -> w822
              disable-tunnel: w798 -> [w888 _]
              frame Disabled {
                n403 = feedback #34(i64 0 ("y")) -> (w890:i64)
                n404 = case "Synchronize trap oscillations - always begin/end with trap 1" shown="1, Default" w888 {
                  tunnel: [w892 w893 w894] -> w891
                  tunnel: w890 -> [w892 w893 _]
                  frame 2 {
                  }
                  frame 3 {
                  }
                  frame 1, Default {
                    n405 = Or(x="Osc traps", y="Initiate trap osc") -> (x .or. y?=w896:bool)
                    n406 = case "Trap sine oscillation (or whatever pattern is stored in memory)" shown="True" w896 {
                      tunnel: [i64 0 ("y") w900] -> w894
                      tunnel: "Initiate trap osc" -> [_ w903]
                      frame False {
                      }
                      frame True {
                        w907 = u16 0
                        w905 = -1
                        n407 = local write "Initiate trap osc"(FALSE ("Initiate trap osc")) -> ()
                        n408 = feedback #35(w907) -> (w909:u16)
                        n409 = Select(t=w907, s=w903, f=w909) -> (s? t:f=w908:u16)
                        n410 = Greater Or Equal?(x=w908, y="Trap osc period (pts)") -> (x >= y?=w914:bool)
                        n411 = Or(x=w903, y=w914) -> (x .or. y?=w915:bool)
                        n412 = Select(t=u16 0, s=w915, f=w908) -> (s? t:f=w899:u16)
                        n413 = feedback #36(w905) -> (w906:i32)
                        n414 = Select(t=w905, s=w903, f=w906) -> (s? t:f=w904:i32)
                        n415 = Increment(x=w904) -> (x+1=w911:i32)
                        n416 = Equal?(x=w899, y=u16 0) -> (x = y?=w912:bool)
                        n417 = Increment(x=w899) -> (x+1=w919:u16)
                        n418 = feedback-in #35(w919) -> ()
                        n419 = Select(t=w911, s=w912, f=w904) -> (s? t:f=w910:i32)
                        n420 = feedback-in #36(w910) -> ()
                        n421 = case shown="False" "Osc trap cont." {
                          tunnel: w910 -> [w923 _]
                          frame False {
                            n422 = Greater Or Equal?(x=w923, y="N trap osc periods") -> (x >= y?=w921:bool)
                            n423 = Not(x=w921) -> (.not. x?=w920:bool)
                            n424 = local write "Osc traps"(w920) -> ()
                          }
                          frame True {
                          }
                        }
                        n425 = xnode ("Memory Read")("Address"=w899, "Memory In"=refnum<k21> "Trap osc memory") -> ("Data"=w900:i64)  [unwired: 1 out]
                      }
                    }
                  }
                }
                n426 = feedback-in #34(w891) -> ()
              }
              frame Enabled {
              }
            }
            n427 = local read "green FB running"() -> (w811:bool)
            n428 = And(x=w811, y="RF synth bd controls green") -> (x .and. y?=w810:bool)
            n429 = case shown="3" w798 {
              tunnel: [w1055 w1303 "BD 1 Frequency 3"] -> w875
              tunnel: [w1095 w1302 w1328] -> w814
              tunnel: ["BD 2 Amplitude 1" "BD 2 Amplitude 2" w1327] -> w806
              tunnel: [w1052 w1299 "BD 1 Amplitude 3"] -> w788
              tunnel: "FB Gains" -> [w1072 w1309 _]
              tunnel: "FB output range" -> [w1073 w1308 _]
              tunnel: w822 -> [w1070 w1306 _]
              tunnel: "BD 2 Frequency 1" -> [w1067 _ _]
              tunnel: "BD 2 Frequency 2" -> [_ w1302 _]
              tunnel: "BD 2 Frequency 3" -> [_ _ w1328]
              tunnel: w810 -> [_ _ w1326]
              tunnel: [w1055 w1300 w1325] -> w779
              tunnel: w778 -> [w1054 w1300 w1325]
              tunnel: [w1039 u64 0 u64 0] -> w777
              tunnel: w776 -> [_ w1295 _]
              frame 1, Default {
                w1086 = fxp<+/-,24,9> 0.0 ("AI1 X Set 2")
                w1080 = u16 0
                w1093 = u64 0 ("f")
                # "Changed by Ronen - correction \nby PID is now implemented not on \nthe Base BD1 frequency but on the last\nfrequency sent."
                # "Added by Ronen -\nUpper and Lower \nLimits for the FB \ngenerated frequency\nto avoid losing bead \nwhen tether breaks"
                # "Explanation of raster scanning:\n1. Cycles: increment counter by 1 every time interlace cycle returns to trap 1. As long as \n  Cycle per Step is larger than counter, keep incrementing counter and do not change step counter.\n  Once counter is equal to Cycles per step, zero counter and increment step counter.\n2. Steps: Increments up every time cycles counter equals cycles per step. Performs the following:\n- To determine DIRECTION of frequency change:  If ScanstepX2 is EQUAL to step counter (full for-back scan finished)\n   frequency increment is set to zero, AND step counter is set to zero. \n   Otherwise: if no change to step counter (because cycleperstep>cycle counter), then no change to frequency\n   increment. \n   If step counter has changed (cycleperstep=cycle counter), then need to figure out direction of frequency change:\n   if step counter is EQUAL to Scansteps: No change to frequency increment\n   Otherwise: If scan steps > step counter - 1 (forward scan NOT completed): increment frequency by 1\n                       If scan steps equal or smaller than step counter -1 (forward scan completed): increment frequency by -1\n\n3. Scans: Increment scan counter every time step counter equals 2Xscan steps (full for-back scan completed)\n    if number of scans > scan counter: Send TRUE to scanning, continue scan\n    if number of scans = scan counter: Send FALSE to Scanning, Scan finished.\n\n  The wire with the asterik can be used as the index for getting the mirror positions in the offset scan."
                # "This signal integration happens no matter what\nso that correct setpoints can be chosen before \nturning on the FB."
                # "Trap 1"
                n430 = local read "AI1 X Set 2"() -> (w1065:fxp<+/-,16,1>)
                n431 = local read "AI1 X Set 1"() -> (w1083:fxp<+/-,16,1>)
                n432 = local read "Scanning"() -> (w1096:bool)
                n433 = Multiply(x=w1065, y="B factor") -> (x*y=w1063:fxp<+/-,48,17>)
                n434 = Or(x=w1096, y="Start scan") -> (x .or. y?=w1050:bool)
                n435 = case shown="True" "Diff FB Measurement?" {
                  tunnel: w1063 -> [w1194 w1203]
                  tunnel: w1083 -> [w1193 w1204]
                  tunnel: [w1191 w1195] -> w1084
                  frame False {
                    n436 = Select(t=w1193, s="Trap Pos FB Monitor T1 or T2", f=w1194) -> (s? t:f=w1191:fxp<+/-,48,17>)
                  }
                  frame True {
                    n437 = Subtract(x=w1204, y=w1203) -> (x-y=w1196:fxp<+/-,48,17>)
                    n438 = Not(x="Negate Diff?") -> (.not. x?=w1202:bool)
                    n439 = Boolean To (0,1)(Boolean="Negate Diff?") -> (0, 1=w1200:i16)
                    n440 = Boolean To (0,1)(Boolean=w1202) -> (0, 1=w1201:i16)
                    n441 = Negate(x=w1200) -> (-x=w1199:i16)
                    n442 = Add(x=w1199, y=w1201) -> (x+y=w1197:i16)
                    n443 = Multiply(x=w1197, y=w1196) -> (x*y=w1195:fxp<+/-,63,32>)
                  }
                }
                n444 = feedback #37(w1080) -> (w1079:u16)
                n445 = Increment(x=w1079) -> (x+1=w1081:u16)
                n446 = Greater Or Equal?(x=w1081, y="Trap Pos FB Int Count") -> (x >= y?=w1053:bool)
                n447 = Select(t=w1080, s=w1053, f=w1081) -> (s? t:f=w1082:u16)
                n448 = feedback-in #37(w1082) -> ()
                n449 = feedback #38(w1086) -> (w1085:fxp<+/-,24,9>)
                n450 = Add(x=w1084, y=w1085) -> (x+y=w1078:fxp<+/-,24,9>)
                n451 = Select(t=w1086, s=w1053, f=w1078) -> (s? t:f=w1089:fxp<+/-,24,9>)
                n452 = feedback-in #38(w1089) -> ()
                n453 = case "Trap 1 X intensity feedback" shown="True" "FB On/Off Set 1" {
                  tunnel: "BD 1 Amplitude 1" -> [w1286 _]
                  tunnel: [w1286 w1290] -> w1052
                  tunnel: w1073 -> [_ w1287]
                  tunnel: w1072 -> [_ w1288]
                  frame False {
                  }
                  frame True {
                    n454 = local read "AI2 Y Sum Set 1"() -> (w1291:i16)
                    n455 = call "Slower PID.vi"("process variable"=w1291, "reset?"="FB Reset Set 1", "setpoint"="FB Setpoint Set 1", "PID gains (x 2^8)"=w1288, "output range"=w1287) -> ("output"=w1292:i16)  [unwired: 10 out]
                    n456 = To Unsigned Word Integer(number=w1292) -> (unsigned 16bit integer=w1290:u16)
                  }
                }
                "BD1 amplitude 1 out" <- w1052
                n457 = Divide(x=w1078, y="Trap Pos FB Int Count") -> (x/y=w1051:fxp<+/-,16,1>)
                n458 = case "For raster scanning" shown="True" w1050 {
                  tunnel: [u64 0 w1134] -> w1042
                  tunnel: [FALSE w1122] -> w1045
                  tunnel: [i16 0 w1121] -> w1046
                  tunnel: w1051 -> [_ w1120]
                  tunnel: "Start scan" -> [_ w1114]
                  frame False {
                    n459 = local write "Scanning"(FALSE ("scanning")) -> ()
                  }
                  frame True {
                    w1128 = u64 0
                    # "Changed by RG, to introduce force\ndependent stopping of the raster scan \nand manual stopping"
                    # "count number of cycles"
                    n460 = feedback #39(w1128) -> (w1131:u64)
                    n461 = Select(t=w1128, s=w1114, f=w1131) -> (s? t:f=w1133:u64)
                    n462 = Increment(x=w1133) -> (x+1=w1126:u64)
                    n463 = Equal?(x=i16 1, y=w1126) -> (x = y?=w1124:bool)
                    n464 = And(x="Abort scan", y=w1124) -> (x .and. y?=w1122:bool)
                    n465 = Greater?(x="Cycles per step", y=w1126) -> (0:w1129:bool)
                    n466 = Select(t=w1126, s=w1129, f=w1128) -> (s? t:f=w1130:u64)
                    n467 = feedback-in #39(w1130) -> ()
                    n468 = Greater?(x=w1120, y="Raster setpoint") -> (0:w1117:bool)
                    n469 = And(x=w1117, y="Raster to target force") -> (x .and. y?=w1115:bool)
                    n470 = case shown="False" w1122 {
                      tunnel: [w1141 i16 0] -> w1134
                      tunnel: w1114 -> [w1166 _]
                      tunnel: w1129 -> [w1159 _]
                      tunnel: w1128 -> [w1149 _]
                      tunnel: [w1143 FALSE] -> w1123
                      tunnel: [w1139 w1177] -> w1121
                      tunnel: [w1142 w1178] -> w1118
                      frame False {
                        w1150 = i64 0
                        # "scan incr."
                        # "freq. incr. mult."
                        # "count steps"
                        n471 = feedback #40(w1149) -> (w1174:u64)
                        n472 = Select(t=w1149, s=w1166, f=w1174) -> (s? t:f=w1142:u64)
                        n473 = Increment(x=w1142) -> (x+1=w1173:u64)
                        n474 = Add(x="Scan steps", y="Scan steps") -> (x+y=w1172:u64)
                        n475 = Select(t=w1142, s=w1159, f=w1173) -> (s? t:f=w1154:u64)
                        n476 = Greater?(x=w1172, y=w1154) -> (0:w1153:bool)
                        n477 = Select(t=w1154, s=w1153, f=w1149) -> (s? t:f=w1170:u64)
                        n478 = feedback-in #40(w1170) -> ()
                        n479 = Equal?(x="Scan steps", y=w1154) -> (x = y?=w1158:bool)
                        n480 = Greater?(x="Scan steps", y=w1142) -> (0:w1169:bool)
                        n481 = feedback #41(w1150) -> (w1171:i64)
                        n482 = Select(t=w1150, s=w1166, f=w1171) -> (s? t:f=w1156:i64)
                        n483 = Increment(x=w1156) -> (x+1=w1168:i64)
                        n484 = Decrement(x=w1156) -> (x-1=w1167:i64)
                        n485 = Select(t=w1168, s=w1169, f=w1167) -> (s? t:f=w1157:i64)
                        n486 = Select(t=w1156, s=w1158, f=w1157) -> (s? t:f=w1155:i64)
                        n487 = Select(t=w1156, s=w1159, f=w1155) -> (s? t:f=w1151:i64)
                        n488 = Select(t=w1151, s=w1153, f=w1150) -> (s? t:f=w1152:i64)
                        n489 = feedback-in #41(w1152) -> ()
                        n490 = feedback #42(w1149) -> (w1165:u64)
                        n491 = Select(t=w1149, s=w1166, f=w1165) -> (s? t:f=w1161:u64)
                        n492 = Increment(x=w1161) -> (x+1=w1162:u64)
                        n493 = Select(t=w1161, s=w1153, f=w1162) -> (s? t:f=w1160:u64)
                        n494 = Greater?(x="Number of scans", y=w1160) -> (0:w1146:bool)
                        n495 = Multiply(x="Scan freq.  increment", y=w1156) -> (x*y=w1141:i64)
                        n496 = Select(t=TRUE, s="Cont. Scan", f=w1146) -> (s? t:f=w1143:bool)
                        n497 = Select(t=w1160, s=w1143, f=w1149) -> (s? t:f=w1163:u64)
                        n498 = feedback-in #42(w1163) -> ()
                        n499 = local read "BD 1 Frequency 1"() -> (w1140:u64)
                        n500 = Increment(x=w1160) -> (x+1=→"Scan I":u64)
                        n501 = Add(x=w1141, y=w1140) -> (x+y=w1139:u64)
                        "Actual Scan freq" <- w1139
                      }
                      frame True {
                        n502 = local read "Actual Scan freq"() -> (w1177:u64)
                        n503 = local read "Scan steps"() -> (w1178:u64)
                      }
                    }
                    "Scanning" <- w1123
                    n504 = case shown="True" w1115 {
                      tunnel: w1118 -> [_ w1138]
                      frame False {
                      }
                      frame True {
                        n505 = Add(x=w1138, y=i16 2) -> (x+y=w1136:u64)
                        n506 = local write "Raster to target force"(FALSE) -> ()
                        n507 = local write "Scan steps"(w1136) -> ()
                      }
                    }
                  }
                }
                n508 = feedback #43(fxp<+/-,24,9> 0.0 ("AI1 X Set 2")) -> (w1090:fxp<+/-,24,9>)
                n509 = Select(t=w1078, s=w1053, f=w1090) -> (s? t:f=w1091:fxp<+/-,24,9>)
                "Trap Pos FB Int Signal" <- w1091
                n510 = feedback-in #43(w1091) -> ()
                n511 = feedback #44(fxp<+/-,16,1> 0.0 ("Trap Pos FB Int-Norm Signal")) -> (w1075:fxp<+/-,16,1>)
                n512 = Select(t=w1051, s=w1053, f=w1075) -> (s? t:f=w1074:fxp<+/-,16,1>)
                "Trap Pos FB Int-Norm Signal" <- w1074
                n513 = feedback-in #44(w1074) -> ()
                n514 = case "For position feedback" shown="True" "Force feedback" {
                  tunnel: [i64 0 w1210] -> w1043
                  tunnel: w1051 -> [_ w1207]
                  tunnel: w1053 -> [_ w1206]
                  frame False {
                  }
                  frame True {
                    n515 = feedback #45(i64 0) -> (w1209:i64)
                    n516 = case shown="True" w1206 {
                      tunnel: [w1211 w1215] -> w1210
                      tunnel: w1209 -> [w1211 _]
                      tunnel: w1207 -> [_ w1214]
                      frame False {
                      }
                      frame True {
                        n517 = xnode ("PID")("process variable"=w1214, "reset?"="Trap Pos. FB Reset", "setpoint"="Trap Pos. FB SP", "PID gains"="Trap Pos. FB Gains", "output range"="Trap pos. FB Range") -> ("output"=w1224:fxp<+/-,16,1>)
                        n518 = Negate(x=w1224) -> (-x=w1223:fxp<+/-,17,2>)
                        n519 = Select(t=w1223, s="Trap Pos FB Negate Action", f=w1224) -> (s? t:f=w1220:fxp<+/-,17,2>)
                        n520 = Scale By Power Of 2(n=u32 15, x=u32 1) -> (x*2^n=w1217:u32)
                        n521 = Multiply(x=w1220, y=w1217) -> (x*y=w1216:fxp<+/-,17,17>)
                        n522 = To Quad Integer(1:w1216) -> (0:w1228:i64)
                        "Trap Pos FB Action" <- w1228
                        n523 = Multiply(x=w1228, y="Trap Pos. FB Mult Factor") -> (x*y=w1226:i64)
                        n524 = Add(x=w1226, y="Trap Pos. FB Offset Factor") -> (x+y=w1215:i64)
                        n525 = disable-structure shown="Disabled" {
                          disable-tunnel: w1215 -> [w1235 _]
                          frame Disabled {
                            w1239 = u32 0
                            n526 = feedback #46() -> (w1236:i64)  [unwired: 1 in]
                            n527 = Add(x=w1235, y=w1236) -> (x+y=w1233:i64)
                            n528 = feedback #47(w1239) -> (w1241:u32)
                            n529 = Increment(x=w1241) -> (x+1=w1230:u32)
                            n530 = Greater Or Equal?(x=w1230, y="FB Trig Integrate") -> (x >= y?=w1231:bool)
                            n531 = Select(t=i64 0, s=w1231, f=w1233) -> (s? t:f=w1237:i64)
                            n532 = feedback-in #46(w1237) -> ()
                            n533 = Select(t=w1239, s=w1231, f=w1230) -> (s? t:f=w1240:u32)
                            n534 = feedback-in #47(w1240) -> ()
                            n535 = And(x=w1231, y="FPGA Trap Trig") -> (x .and. y?=w1238:bool)
                            n536 = case "Trap FB trigger excitation laser ON" shown="True" w1238 {
                              tunnel: w1233 -> [_ w1245]
                              tunnel: w1230 -> [_ w1243]
                              frame False {
                              }
                              frame True {
                                n537 = Not(x="TTrig Negate Pos") -> (.not. x?=w1252:bool)
                                n538 = Boolean To (0,1)(Boolean="TTrig Negate Pos") -> (0, 1=w1250:i16)
                                n539 = Boolean To (0,1)(Boolean=w1252) -> (0, 1=w1251:i16)
                                n540 = Negate(x=w1250) -> (-x=w1249:i16)
                                n541 = Add(x=w1249, y=w1251) -> (x+y=w1248:i16)
                                n542 = Multiply(x=w1248, y=w1245) -> (x*y=w1247:i64)
                                "TTrig Sig" <- w1247
                                n543 = Multiply(x="FPGA TTrig Thresh", y=w1243) -> (x*y=w1244:i64)
                                "TTrig Fin Thresh" <- w1244
                                n544 = Greater Or Equal?(x=w1247, y=w1244) -> (x >= y?=w1246:bool)
                                n545 = case shown="True" w1246 {
                                frame False {
                                }
                                frame True {
                                w1255 = TRUE ("Green FB On/Off")
                                w1257 = u8 2 ("Operating Mode")
                                n546 = local write "Operating Mode"(w1257) -> ()
                                n547 = local write item#-1(w1257) -> ()
                                n548 = local write item#-1(w1255) -> ()
                                n549 = local write "FPGA Trap Trig"(FALSE ("FPGA Trap Trig")) -> ()
                                "TTrig?" <- w1255
                                }
                                }
                              }
                            }
                          }
                          frame Enabled {
                          }
                        }
                      }
                    }
                    n550 = feedback-in #45(w1210) -> ()
                  }
                }
                n551 = case shown="True" "Symmetric FB/Raster" {
                  tunnel: [w1100 w1104] -> w1041
                  tunnel: w1043 -> [w1100 w1105]
                  tunnel: w1042 -> [w1099 w1102]
                  tunnel: [w1099 w1101] -> w1040
                  frame False {
                  }
                  frame True {
                    n552 = Scale By Power Of 2(n=i16 -1, x=w1105) -> (x*2^n=w1104:i64)
                    n553 = Scale By Power Of 2(n=i16 -1, x=w1102) -> (x*2^n=w1101:u64)
                  }
                }
                n554 = Add(x=w1041, y=w1040) -> (x+y=w1039:u64)
                n555 = And(x="Force feedback", y="Dynamic Force FB (Ronen)") -> (x .and. y?=w1060:bool)
                n556 = case shown="True" w1060 {
                  tunnel: w1041 -> [w1182 w1186]
                  tunnel: [w1181 w1185] -> w1047
                  tunnel: w1054 -> [_ w1184]
                  tunnel: w1053 -> [_ w1183]
                  frame False {
                    # "(BD1 Frequency 1)"
                    n557 = Add(x="BD 1 Frequency 1", y=w1182) -> (x+y=w1181:u64)
                  }
                  frame True {
                    n558 = case shown="True" w1183 {
                      tunnel: w1186 -> [_ w1190]
                      tunnel: [w1187 w1189] -> w1185
                      tunnel: w1184 -> [w1187 w1188]
                      frame False {
                      }
                      frame True {
                        n559 = Add(x=w1188, y=w1190) -> (x+y=w1189:u64)
                      }
                    }
                  }
                }
                n560 = case shown="True" w1045 {
                  tunnel: [w1107 w1109] -> w1048
                  tunnel: w1047 -> [w1107 _]
                  tunnel: w1046 -> [_ w1109]
                  frame False {
                  }
                  frame True {
                    n561 = local write "BD 1 Frequency 1"(w1109) -> ()
                    n562 = local write "Abort scan"(FALSE) -> ()
                  }
                }
                n563 = Select(t=w1070, s="Trap 1 osc enable", f=i64 0) -> (s? t:f=w1068:i64)
                n564 = Select(t=w1093, s="Scan BD", f=w1040) -> (s? t:f=w1092:u64)
                n565 = Select(t=w1040, s="Scan BD", f=w1093) -> (s? t:f=w1059:u64)
                n566 = Add(x=w1092, y=w1067) -> (x+y=w1095:u64)
                n567 = Compound Arithmetic op=ADD(w1068, w1048, w1059) -> (w1058:u64)
                n568 = In Range and Coerce(upper limit="FB Max Frequency", x=w1058, lower limit="FB Min frequency") -> (coerced(x)=w1055:u64)  [unwired: 1 out]
                "BD1 Frequency Out 1" <- w1055
              }
              frame 2 {
                # "Trap 2"
                n569 = local read "Symmetric FB/Raster"() -> (w1298:bool)
                n570 = case shown="True" w1298 {
                  tunnel: "BD 1 Frequency 2" -> [w1312 w1315]
                  tunnel: [w1312 w1314] -> w1296
                  tunnel: w1295 -> [_ w1313]
                  frame False {
                  }
                  frame True {
                    n571 = Subtract(x=w1315, y=w1313) -> (x-y=w1314:u64)
                  }
                }
                n572 = case "Trap 2 X intensity feedback" shown="True" "FB On/Off Set 2" {
                  tunnel: [w1316 w1319] -> w1299
                  tunnel: "BD 1 Amplitude 2" -> [w1316 _]
                  tunnel: w1309 -> [_ w1318]
                  tunnel: w1308 -> [_ w1317]
                  frame False {
                  }
                  frame True {
                    n573 = local read "AI2 Y Sum Set 2"() -> (w1322:i16)
                    n574 = call "Slower PID.vi"("process variable"=w1322, "reset?"="FB Reset Set 2", "setpoint"="FB Setpoint Set 2", "PID gains (x 2^8)"=w1318, "output range"=w1317) -> ("output"=w1320:i16)  [unwired: 10 out]
                    n575 = To Unsigned Word Integer(number=w1320) -> (unsigned 16bit integer=w1319:u16)
                  }
                }
                "BD1 amplitude 2 out" <- w1299
                n576 = Select(t=w1306, s="Trap 2 osc enable", f=i64 0) -> (s? t:f=w1305:i64)
                n577 = Add(x=w1296, y=w1305) -> (x+y=w1303:u64)
                "BD1 Frequency Out 2" <- w1303
              }
              frame 3 {
                # "Fluorescence period"
                n578 = disable-structure shown="Disabled" {
                  disable-tunnel: [w1336 _] -> w1327
                  disable-tunnel: w1326 -> [w1335 _]
                  frame Disabled {
                    # "Remember if FB was previously on/off"
                    n579 = feedback #48(FALSE) -> (w1331:bool)
                    n580 = case shown="True" w1335 {
                      tunnel: [w1338 w1354] -> w1336
                      tunnel: "BD 2 Amplitude 3" -> [w1338 _]
                      tunnel: [FALSE TRUE] -> w1332
                      tunnel: w1331 -> [_ w1340]
                      frame False {
                      }
                      frame True {
                        # "Makes it so first time FB run when turned on, the PID sees the detector intensity from the last time FB was running, rather than something near zero. Especially assuming the setpoint is not changing, this will make the FB more stable when resuming, and not overshoot the turnon intensity."
                        # "FB output range: 0 should be low, full scale is 12 bits.\nBut be careful not to go over, then higher bits just get ignored by RF board, so output will actually jump down and be unstable. Keep it under 4000 to be safe."
                        n581 = local read "Green FB Sum"() -> (w1339:i16)
                        n582 = feedback-in #49(w1339) -> ()
                        n583 = feedback #49(i16 0 ("Green FB Sum")) -> (w1342:i16)
                        n584 = Select(t=w1339, s=w1340, f=w1342) -> (s? t:f=w1341:i16)
                        n585 = Bundle("P3 2"="P3 2", "I3 2"="I3 2", "D3 2"="D3 2") -> (w1353:cluster{"P3 2":i16, "I3 2":i16, "D3 2":i16})  [unwired: 1 in]
                        n586 = Bundle("RF synth green feedback max"="RF synth green feedback max", i16 0) -> (w1345:cluster{"RF synth green feedback max":i16, i16})  [unwired: 1 in]
                        n587 = call "Slower PID.vi"("process variable"=w1341, "reset?"="Green FB Reset 2", "setpoint"="Green FB Setpoint 2", "PID gains (x 2^8)"=w1353, "output range"=w1345) -> ("output"=w1355:i16)  [unwired: 10 out]
                        n588 = To Unsigned Word Integer(number=w1355) -> (unsigned 16bit integer=w1354:u16)
                      }
                    }
                    n589 = feedback-in #48(w1332) -> ()
                  }
                  frame Enabled {
                  }
                }
              }
            }
            n590 = Split Number(x=w875) -> (hi(x)=w874:u32, lo(x)=w873:u32)
            n591 = Boolean To (0,1)(Boolean="+ phase (DIO)") -> (0, 1=w835:i16)
            n592 = Split Number(x=w874) -> (lo(x)=w872:u16)  [unwired: 1 out]
            n593 = Split Number(x=w873) -> (hi(x)=w871:u16, lo(x)=w870:u16)
            n594 = Split Number(x=w872) -> (hi(x)=w864:u8, lo(x)=w863:u8)
            n595 = Split Number(x=w871) -> (hi(x)=w862:u8, lo(x)=w861:u8)
            n596 = Split Number(x=w870) -> (hi(x)=w860:u8, lo(x)=w859:u8)
            n597 = Multiply(x=w835, y="Phase count adjustment (DIO)") -> (x*y=w831:i16)
            n598 = feedback #50(TRUE) -> (w820:bool)
            n599 = Not(x=w820) -> (.not. x?=w819:bool)
            n600 = feedback-in #50(w819) -> ()
            n601 = feedback #51(i16 0) -> (w833:i16)
            n602 = Subtract(x=w833, y=w831) -> (x-y=w832:i16)
            "DIO Relative phase" <- w832
            n603 = feedback-in #51(w832) -> ()
            n604 = Add(x=w838, y=w831) -> (x+y=w837:u32)
            n605 = Build Array "BD 1 nu Stack"(w864, w863, w862, w861, w860, w859) -> (w858:u8[])
            n606 = Not Equal?(x=w798, y=u8 3) -> (x != y?=w807:bool)
            n607 = case "Store in RF board F1 or F2" shown="True" w819 {
              tunnel: [w1030 w1034] -> w849
              tunnel: [u8 10 u8 4] -> w850
              tunnel: "Swap F1 and F2" -> [w1031 w1034]
              tunnel: "BD 2 Frequency 1" -> [_ w1033]
              tunnel: "BD 2 Frequency 2" -> [w1029 _]
              tunnel: [w1029 w1033] -> w815
              frame False {
                # "for RF synth controls\ngreen: F1/F2 stay same"
                # "F2 address (hex)"
                n608 = Not(x=w1031) -> (.not. x?=w1030:bool)
              }
              frame True {
                # "low chooses F1"
                # "F1 address (hex)"
              }
            }
            n609 = Select(t=w815, s="RF synth bd controls green", f=w814) -> (s? t:f=w813:u64)
            n610 = Split Number(x=w813) -> (hi(x)=w869:u32, lo(x)=w868:u32)
            n611 = Split Number(x=w869) -> (lo(x)=w867:u16)  [unwired: 1 out]
            n612 = Split Number(x=w868) -> (hi(x)=w866:u16, lo(x)=w865:u16)
            n613 = Split Number(x=w867) -> (hi(x)=w857:u8, lo(x)=w856:u8)
            n614 = Split Number(x=w866) -> (hi(x)=w855:u8, lo(x)=w854:u8)
            n615 = Split Number(x=w865) -> (hi(x)=w853:u8, lo(x)=w852:u8)
            n616 = feedback #52(u16 0 ("BD 2 Amplitude 3")) -> (w804:u16)
            n617 = Select(t=w804, s=w807, f=w806) -> (s? t:f=w805:u16)
            n618 = feedback-in #52(w805) -> ()
            n619 = And(x=w807, y=w810) -> (x .and. y?=w809:bool)
            n620 = Build Array "BD 2 nu Stack"(w857, w856, w855, w854, w853, w852) -> (w851:u8[])
            n621 = Select(t=w804, s=w809, f=w806) -> (s? t:f=w787:u16)
            n622 = flat-sequence "Update trap RF synth board settings to be used for the upcoming trap cycle." {
              tunnel: w851 -> [w978]
              tunnel: w858 -> [w979]
              tunnel: [w979] -> w802
              tunnel: [w978] -> w801
              tunnel: w850 -> [w980]
              tunnel: w802 -> [w982]
              tunnel: w801 -> [w981]
              tunnel: w789 -> [w993]
              tunnel: w791 -> [w992]
              tunnel: w790 -> [w991]
              frame #0 {
                # "To possibly delay\nthese writes to very\nend of loop (for x and\ny phase adjust)"
                n623 = call "Wait8"("Count(Ticks)"="Next trap write delay (ticks)") -> ()  [unwired: 1 out]
              }
              frame #1 {
                # "Next trap RF frequency:\n\nWrite next trap cycle frequency to buffer."
                n624 = for {
                  tunnel: w982 -> [w988] mode=indexing
                  tunnel: w981 -> [w987] mode=indexing
                  tunnel: w980 -> [w985]
                  i -> [w986]
                  n625 = To Unsigned Byte Integer(number=w986) -> (unsigned 8bit integer=w983:u8)
                  n626 = Add(x=w985, y=w983) -> (x+y=w984:u8)
                  n627 = call "write to RF synth bd.vi"("Address Byte"=w984, "BD 2 Byte"=w987, "BD 1 Byte"=w988) -> ()
                }
              }
              frame #2 {
                w989 = TRUE ("Connector1/DIO15")
                # "Send udclk high\n(BD 1 and 2) to make the new frequency active in F1 or F2 word. But it won't actually be the used frequency until FSK switches to it (begining of next cycle)."
                n628 = xnode "FPGA I/O Node"("Connector1/DIO30"=w989, "Connector1/DIO29"=w989) -> ()  [unwired: 2 in, 2 out]
              }
              frame #3 {
                w990 = FALSE ("Connector1/DIO15")
                n629 = xnode "FPGA I/O Node"("Connector1/DIO30"=w990, "Connector1/DIO29"=w990) -> ()  [unwired: 2 in, 2 out]
              }
              frame #4 {
                # "Next trap RF phase offset:\n\nSet the next trap cycle amplitude to the buffer. Won't become active until udclk is set high at proper time at the begining of the next cycle."
                n630 = case shown="True" w993 {
                  tunnel: w992 -> [_ w994]
                  tunnel: w991 -> [_ w995]
                  frame False {
                  }
                  frame True {
                    # "phase 1 address start"
                    n631 = for {
                      tunnel: w994 -> [w1002] mode=indexing
                      tunnel: w995 -> [w1001] mode=indexing
                      tunnel: u8 0 -> [w999]
                      i -> [w1000]
                      n632 = To Unsigned Byte Integer(number=w1000) -> (unsigned 8bit integer=w997:u8)
                      n633 = Add(x=w999, y=w997) -> (x+y=w998:u8)
                      n634 = call "write to RF synth bd.vi"("Address Byte"=w998, "BD 2 Byte"=w1001, "BD 1 Byte"=w1002) -> ()
                    }
                  }
                }
              }
              frame #5 {
                # "Prep to reset RF phase to zero at start of next cycle. Only reset BD 1. Do nothing to BD 2. This puts the settings in the buffer. A udclk high will make both this phase reset and possibly a new phase offset setting active."
                n635 = case shown="True" "RF phase reset before cycles" {
                  frame False {
                  }
                  frame True {
                    w1005 = u8 66  # BD 1 reset
                    n636 = call "write to RF synth bd.vi"("Address Byte"=u8 31, "BD 2 Byte"=u8 2, "BD 1 Byte"=w1005) -> ()
                  }
                }
              }
              frame #6 {
                # "Address"
                # "Data BD 2"
                # "Data BD 1"
                # "If phase reset wasn't chosen previously, these actions will have no affect. For both BD's, data should be binary 10, and address should be hex 1F (bin 01 1111)"
                # "This sets up the digital communication lines to restart phase accumulation (start RF running agin). It cancels out the possible phase reset. Just need to set WR DIO low then udclk DIOhigh  to make this happen. Doing this here early (and not using the usual board write function) speeds things up.\n\nRestarts RF (BD 1 only, BD2 never stopped in first place)."
                n637 = xnode "FPGA I/O Node"("Connector1/DIO0"=FALSE, "Connector1/DIO1"=FALSE, "Connector1/DIO2"=FALSE, "Connector1/DIO3"=FALSE, "Connector1/DIO4"=FALSE, "Connector1/DIO5"=FALSE, "Connector1/DIO6"=TRUE, "Connector1/DIO7"=FALSE, "Connector1/DIO8"=FALSE, "Connector1/DIO9"=TRUE, "Connector1/DIO10"=TRUE, "Connector1/DIO11"=TRUE, "Connector1/DIO12"=TRUE, "Connector1/DIO13"=TRUE, "Connector1/DIO20"=FALSE, "Connector1/DIO21"=FALSE, "Connector1/DIO22"=FALSE, "Connector1/DIO23"=FALSE, "Connector1/DIO24"=FALSE, "Connector1/DIO25"=FALSE, "Connector1/DIO26"=TRUE, "Connector1/DIO27"=FALSE) -> ()  [unwired: 22 in, 22 out]
              }
            }
            n638 = feedback #53(fxp<+,8,8> 0.0) -> (w784:fxp<+,8,8>)
            n639 = Increment(x=w784) -> (x+1=w782:fxp<+,8,8>)
            n640 = feedback-in #53(w782) -> ()
            n641 = case "Trap RF phase offset control methods" shown="3" "Phase offset method" {
              tunnel: [fxp<+,14,14> 0.0 ("Phase BD 1") w928 w943 w972] -> w792
              tunnel: "Phase Trap 1" -> [_ w929 w944 _]
              tunnel: w798 -> [_ w930 w945 w973]
              tunnel: [FALSE TRUE TRUE TRUE] -> w789
              tunnel: "Phase Trap 2" -> [_ w926 w941 _]
              tunnel: w782 -> [_ _ w940 _]
              frame 0, Default {
              }
              frame 1 {
                # "Constant increment of phase offset with each trap cycle. This results in a constant phase difference between trap cycles. \nOnly for traps 1 and 2 (set phase offset to zero for set three)."
                n642 = case shown="1, Default" w930 {
                  tunnel: w929 -> [_ _ w936]
                  tunnel: [w932 fxp<+,14,14> 0.0 w937] -> w928
                  tunnel: w926 -> [w931 _ _]
                  frame 2 {
                    n643 = feedback #54(fxp<+,14,14> 0.0) -> (w934:fxp<+,14,14>)
                    n644 = Add(x=w931, y=w934) -> (x+y=w932:fxp<+,14,14>)
                    n645 = feedback-in #54(w932) -> ()
                  }
                  frame 3 {
                  }
                  frame 1, Default {
                    n646 = feedback #55(fxp<+,14,14> 0.0) -> (w939:fxp<+,14,14>)
                    n647 = Add(x=w936, y=w939) -> (x+y=w937:fxp<+,14,14>)
                    n648 = feedback-in #55(w937) -> ()
                  }
                }
              }
              frame 2 {
                # "Changing increment of phase offset with each trap cycle. This results in a constant change in phase difference between trap cycles. \nOnly for traps 1 and 2 (set phase offset to zero for set three)."
                n649 = case shown="2" w945 {
                  tunnel: w944 -> [_ _ w955]
                  tunnel: [w946 fxp<+,14,14> 0.0 w953] -> w943
                  tunnel: w941 -> [w948 _ _]
                  tunnel: w940 -> [w949 _ w956]
                  frame 2 {
                    n650 = Multiply(x=w948, y=w949) -> (x*y=w947:fxp<+,16,16>)
                    n651 = feedback #56(fxp<+,14,14> 0.0) -> (w951:fxp<+,14,14>)
                    n652 = Add(x=w947, y=w951) -> (x+y=w946:fxp<+,14,14>)
                    n653 = feedback-in #56(w946) -> ()
                  }
                  frame 3 {
                  }
                  frame 1, Default {
                    n654 = Multiply(x=w955, y=w956) -> (x*y=w954:fxp<+,16,16>)
                    n655 = feedback #57(fxp<+,14,14> 0.0) -> (w958:fxp<+,14,14>)
                    n656 = Add(x=w954, y=w958) -> (x+y=w953:fxp<+,14,14>)
                    n657 = feedback-in #57(w953) -> ()
                  }
                }
              }
              frame 3 {
                w965 = u32 1013904223  # LCG constant C (add)
                w967 = fxp<+,21,21> 1664525.0  # LCG constant A (multiply)
                # "Set a random phase offset. Random number generated using the LCG method. Constants and method taken from NI white noise generator code (method is general though)."
                # "shift to 14 significant bits"
                n658 = feedback #58(u32 4294967295 ("seed")) -> (w962:u32)
                n659 = Multiply(x=w962, y=w967) -> (x*y=w966:u32)
                n660 = Split Number(x=w962) -> (hi(x)=w968:u16)  [unwired: 1 out]
                n661 = To Unsigned Word Integer(number=w968) -> (unsigned 16bit integer=w960:u16)
                n662 = Add(x=w966, y=w965) -> (x+y=w964:fxp<+,32,32>)
                n663 = To Unsigned Long Integer(number=w964) -> (unsigned 32bit integer=w961:u32)
                n664 = feedback-in #58(w961) -> ()
                n665 = Scale By Power Of 2(n=i8 -2 ("Uniform scale factor"), x=w960) -> (x*2^n=w969:u16)
                n666 = To Fixed-Point(number=w969) -> (fixed-point=w959:fxp<+,14,14>)  [unwired: 1 in]
                "Random phase generated" <- w959
                n667 = case shown="1, Default" w973 {
                  tunnel: [w974 fxp<+,14,14> 0.0 w976] -> w972
                  tunnel: w959 -> [w974 _ w976]
                  frame 2 {
                  }
                  frame 3 {
                  }
                  frame 1, Default {
                  }
                }
              }
            }
            n668 = To Unsigned Word Integer(number=w792) -> (unsigned 16bit integer=w797:u16)
            n669 = Split Number(x=w797) -> (hi(x)=w795:u8, lo(x)=w796:u8)
            n670 = Split Number(x=u16 0) -> (hi(x)=w793:u8, lo(x)=w794:u8)
            n671 = Build Array ("BD 1 A Stack")(w795, w796) -> (w791:u8[])
            n672 = Build Array ("BD 1 A Stack")(w793, w794) -> (w790:u8[])
          }
        }
      }
    }
  }
  n673 = while "532 nm green fluorescent laser interlacing (DO to IA 532 nm AOM ME amp)." {
    shift-right: [w1359] -> _
    shift-left: w3 -> [w1364]
    shift-right: [w1358] -> _
    shift-left: w4 -> [w1356]
    stop <- FALSE stop-if-true
    n674 = flat-sequence {
      tunnel: w1364 -> [w1367]
      tunnel: [w1366] -> w1362
      tunnel: [w1367] -> w1360
      tunnel: [w1368] -> w1357
      tunnel: w1356 -> [w1368]
      tunnel: [w1371] -> w1363
      tunnel: w1362 -> [w1371]
      tunnel: [w1370] -> w1361
      tunnel: w1360 -> [w1370]
      tunnel: w1357 -> [w1369]
      tunnel: [w1383] -> w1359
      tunnel: w1363 -> [w1402]
      tunnel: w1361 -> [w1399]
      tunnel: [w1372] -> w1358
      frame #0 {
        n675 = call "Loop Timer9"("Count(Ticks)"=w1367) -> ("Tick Count(Ticks)"=w1366:u32)
      }
      frame #1 {
        # "Then to PRL 440 amp\nOR to RF synth board FSK in"
        n676 = xnode "FPGA I/O Node"("Connector1/DIO37"=w1369, "Connector1/DIO38"=w1369, "Connector1/DIO39"=w1369, "Connector1/DIO26"=w1369, "Connector1/DIO27"=w1369, "Connector1/DIO32"=w1369) -> ()  [unwired: 6 in, 6 out]
      }
      frame #2 {
        n677 = feedback-in #59(w1402) -> ()
        n678 = feedback #59(w1402) -> (w1401:u32)
        n679 = Subtract(x=w1402, y=w1401) -> (x-y=w1400:u32)
        n680 = Subtract(x=w1400, y=w1399) -> (x-y=w1376:u32)
        n681 = Number To Boolean Array(number=w1376) -> (Boolean array=w1377:bool[])
        n682 = Or Array Elements(Boolean array=w1377) -> (logical OR=w1375:bool)
        n683 = Boolean To (0,1)(Boolean="+ phase (GI)") -> (0, 1=w1388:i16)
        n684 = Boolean To (0,1)(Boolean=w1375) -> (0, 1=w1382:i16)
        n685 = To Unsigned Byte Integer(number=w1382) -> (unsigned 8bit integer=w1379:u8)
        n686 = Multiply(x=w1388, y="Phase count adjustment (GI)") -> (x*y=w1385:i16)
        n687 = feedback #60(u8 0) -> (w1380:u8)
        n688 = Add(x=w1379, y=w1380) -> (x+y=w1378:u8)
        "GI Late Counter" <- w1378
        n689 = feedback-in #60(w1378) -> ()
        n690 = feedback #61(i16 0) -> (w1386:i16)
        n691 = Subtract(x=w1386, y=w1385) -> (x-y=w1384:i16)
        "GI Relative phase" <- w1384
        n692 = feedback-in #61(w1384) -> ()
        n693 = feedback #62(TRUE) -> (w1394:bool)
        n694 = case shown="2" "Operating Mode" {
          tunnel: [TRUE FALSE w1427] -> w1373
          tunnel: w1394 -> [_ _ w1424]
          frame 0, Default {
          }
          frame 1 {
          }
          frame 2 {
            n695 = Not(x=w1424) -> (.not. x?=w1426:bool)
            n696 = Select(t=w1426, s="Invert GI", f=w1424) -> (s? t:f=w1427:bool)
          }
        }
        n697 = Not(x=w1394) -> (.not. x?=w1391:bool)
        n698 = Select(t="Green interlace ON count", s=w1391, f="Green interlace OFF count") -> (s? t:f=w1396:u16)
        n699 = Subtract(x=w1396, y=w1376) -> (x-y=w1389:u32)
        n700 = Add(x=w1389, y=w1385) -> (x+y=w1383:u32)
        n701 = feedback-in #62(w1391) -> ()
        n702 = case shown="True" "Green long-scale interlacing" {
          tunnel: w1373 -> [w1403 w1411]
          tunnel: [w1403 w1412] -> w1372
          frame False {
          }
          frame True {
            n703 = feedback #63(i16 1) -> (w1418:i16)
            n704 = Increment(x=w1418) -> (x+1=w1417:i16)
            n705 = feedback #64("Number of ON cycles") -> (w1404:i16)
            n706 = Greater?(x=w1404, y=w1418) -> (0:w1413:bool)
            n707 = Select(t=w1417, s=w1413, f=i16 1) -> (s? t:f=w1415:i16)
            n708 = feedback-in #63(w1415) -> ()
            n709 = feedback #65(TRUE) -> (w1410:bool)
            n710 = Not(x=w1410) -> (.not. x?=w1409:bool)
            n711 = Select(t=w1410, s=w1413, f=w1409) -> (s? t:f=w1408:bool)
            n712 = Select(t="Number of ON cycles", s=w1408, f="Number of OFF cycles") -> (s? t:f=w1406:i16)
            n713 = feedback-in #64(w1406) -> ()
            n714 = feedback-in #65(w1408) -> ()
            n715 = case shown="False" w1408 {
              tunnel: [FALSE w1421] -> w1412
              tunnel: w1411 -> [_ w1421]
              frame False {
              }
              frame True {
              }
            }
          }
        }
      }
    }
  }
  n716 = while "Green excitation laser feedback measurement" {
    shift-right: [w1428] -> _
    shift-left: w3 -> [w1433]
    stop <- FALSE stop-if-true
    n717 = flat-sequence {
      tunnel: w1433 -> [w1435]
      tunnel: [w1436] -> w1431
      tunnel: [w1435] -> w1429
      tunnel: [w1443] -> w1432
      tunnel: w1431 -> [w1443]
      tunnel: [w1442] -> w1430
      tunnel: w1429 -> [w1442]
      tunnel: [w1455] -> w1428
      tunnel: w1432 -> [w1466]
      tunnel: w1430 -> [w1463]
      frame #0 {
        n718 = call "Loop Timer6"("Count(Ticks)"=w1435) -> ("Tick Count(Ticks)"=w1436:u32)
      }
      frame #1 {
        n719 = xnode "FPGA I/O Node"("Connector1/DIO35"=TRUE) -> ("Chassis2/Mod2/AI0"=w1441:i16, "Chassis2/Mod2/AI1"=w1440:i16, "Chassis2/Mod2/AI2"=w1437:i16)  [unwired: 4 in, 4 out]
        "Green FB Sum" <- w1437
        n720 = Bundle("Chassis2/Mod2/AI0"=w1441, "Chassis2/Mod2/AI1"=w1440, "Chassis2/Mod2/AI2"=w1437) -> (→"Green FB Signals":T10)  [unwired: 1 out]
      }
      frame #2 {
        n721 = feedback-in #66(w1466) -> ()
        n722 = feedback #66(w1466) -> (w1465:u32)
        n723 = Subtract(x=w1466, y=w1465) -> (x-y=w1464:u32)
        n724 = xnode "FPGA I/O Node"("Connector1/DIO35"=FALSE) -> ()  [unwired: 1 in, 1 out]
        n725 = Subtract(x=w1464, y=w1463) -> (x-y=w1445:u32)
        n726 = Subtract(x="Green FB Count", y=w1445) -> (x-y=w1459:u32)
        n727 = Number To Boolean Array(number=w1445) -> (Boolean array=w1446:bool[])
        n728 = Or Array Elements(Boolean array=w1446) -> (logical OR=w1444:bool)
        "Green FB Late?" <- w1444
        n729 = Boolean To (0,1)(Boolean="+ phase (Green FB)") -> (0, 1=w1457:i16)
        n730 = Boolean To (0,1)(Boolean=w1444) -> (0, 1=w1451:i16)
        n731 = Multiply(x=w1457, y="Phase count adjustment (Green FB)") -> (x*y=w1452:i16)
        n732 = Add(x=w1459, y=w1452) -> (x+y=w1455:u32)
        n733 = To Unsigned Word Integer(number=w1451) -> (unsigned 16bit integer=w1448:u16)
        n734 = feedback #67(i16 0) -> (w1454:i16)
        n735 = Subtract(x=w1454, y=w1452) -> (x-y=w1453:i16)
        "Green FB Relative Phase" <- w1453
        n736 = feedback-in #67(w1453) -> ()
        n737 = feedback #68(u16 0) -> (w1449:u16)
        n738 = Add(x=w1448, y=w1449) -> (x+y=w1447:u16)
        "Green Late Counter" <- w1447
        n739 = feedback-in #68(w1447) -> ()
      }
    }
  }
  n740 = while "Control APD data integration - stream to host" {
    shift-right: [w1469] -> _
    shift-left: w6 -> [w1474]
    stop <- FALSE stop-if-true
    n741 = flat-sequence {
      tunnel: w1474 -> [w1476]
      tunnel: [w1477] -> w1472
      tunnel: [w1476] -> w1470
      tunnel: [w1485] -> w1473
      tunnel: w1472 -> [w1485]
      tunnel: [w1484] -> w1471
      tunnel: w1470 -> [w1484]
      tunnel: [w1483] -> w1468
      tunnel: [w1482] -> w1467
      tunnel: [w1519] -> w1469
      tunnel: w1473 -> [w1531]
      tunnel: w1471 -> [w1528]
      tunnel: w1468 -> [w1512]
      tunnel: w1467 -> [w1511]
      frame #0 {
        n742 = call "Loop Timer4"("Count(Ticks)"=w1476) -> ("Tick Count(Ticks)"=w1477:u32)
      }
      frame #1 {
        n743 = flat-sequence {
          tunnel: [w1487] -> w1481
          tunnel: w1481 -> [w1489]
          tunnel: [w1491] -> w1480
          tunnel: [w1490] -> w1479
          tunnel: [w1489] -> w1478
          tunnel: [w1497] -> w1482
          tunnel: [w1498] -> w1483
          tunnel: w1480 -> [w1498]
          tunnel: w1479 -> [w1497]
          tunnel: w1478 -> [w1496]
          frame #0 {
            # "use two separate variable so each APD won't\nhave to wait to read"
            n744 = feedback #69(FALSE) -> (w1486:bool)
            "APD1 out state" <- w1486
            "APD2 out state" <- w1486
            n745 = Not(x=w1486) -> (.not. x?=w1487:bool)
            n746 = feedback-in #69(w1487) -> ()
          }
          frame #1 {
            n747 = local read "APD 1 Counts 1"() -> (w1495:u32)
            n748 = local read "APD 1 Counts 0"() -> (w1494:u32)
            n749 = local read "APD 2 Counts 1"() -> (w1493:u32)
            n750 = local read "APD 2 Counts 0"() -> (w1492:u32)
            n751 = Select(t=w1495, s=w1489, f=w1494) -> (s? t:f=w1491:u32)
            n752 = Select(t=w1493, s=w1489, f=w1492) -> (s? t:f=w1490:u32)
          }
          frame #2 {
            n753 = case shown="True" w1496 {
              frame False {
                w1499 = u32 0 ("APD 1 Counts 0")
                n754 = local write "APD 1 Counts 0"(w1499) -> ()
                n755 = local write "APD 2 Counts 0"(w1499) -> ()
              }
              frame True {
                w1500 = u32 0 ("APD 1 Counts 1")
                n756 = local write "APD 1 Counts 1"(w1500) -> ()
                n757 = local write "APD 2 Counts 1"(w1500) -> ()
              }
            }
          }
        }
      }
      frame #2 {
        n758 = feedback-in #70(w1531) -> ()
        n759 = feedback #70(w1531) -> (w1530:u32)
        n760 = Subtract(x=w1531, y=w1530) -> (x-y=w1529:u32)
        n761 = Subtract(x=w1529, y=w1528) -> (x-y=w1504:u32)
        n762 = case shown="True" "APD to FIFO" {
          tunnel: w1512 -> [_ w1534]
          tunnel: w1511 -> [_ w1532]
          frame False {
          }
          frame True {
            n763 = flat-sequence {
              tunnel: 0 ("Timeout") -> [w1536]
              tunnel: w1534 -> [w1537]
              tunnel: [w1536] -> w1533
              tunnel: w1533 -> [w1539]
              tunnel: w1532 -> [w1538]
              frame #0 {
                n764 = xnode ("FIFO Write")("Element"=w1537, "Timeout"=w1536) -> ()  [unwired: 1 in, 2 out]
              }
              frame #1 {
                n765 = xnode ("FIFO Write")("Element"=w1538, "Timeout"=w1539) -> ()  [unwired: 1 in, 2 out]
              }
            }
          }
        }
        n766 = Subtract(x="APD Acq Rate Count", y=w1504) -> (x-y=w1520:u32)
        n767 = Number To Boolean Array(number=w1504) -> (Boolean array=w1505:bool[])
        n768 = Or Array Elements(Boolean array=w1505) -> (logical OR=w1503:bool)
        "APD Acq Late?" <- w1503
        n769 = Boolean To (0,1)(Boolean=w1503) -> (0, 1=w1510:i16)
        n770 = To Unsigned Word Integer(number=w1510) -> (unsigned 16bit integer=w1507:u16)
        n771 = Boolean To (0,1)(Boolean="+ phase (APD Acq)") -> (0, 1=w1516:i16)
        n772 = feedback #71(u16 0) -> (w1508:u16)
        n773 = Add(x=w1507, y=w1508) -> (x+y=w1506:u16)
        "APD Acq Late Counter" <- w1506
        n774 = feedback-in #71(w1506) -> ()
        n775 = Multiply(x=w1516, y="Phase Count Adjustment (APD Acq)") -> (x*y=w1513:i16)
        n776 = Add(x=w1520, y=w1513) -> (x+y=w1519:u32)
        n777 = feedback #72(i16 0) -> (w1518:i16)
        n778 = Subtract(x=w1518, y=w1513) -> (x-y=w1515:i16)
        "APD Acq Relative Phase" <- w1515
        n779 = feedback-in #72(w1515) -> ()
        n780 = To Word Integer(number=w1512) -> (16bit integer=w1521:i16)
        n781 = To Word Integer(number=w1511) -> (16bit integer=w1522:i16)
        n782 = Multiply(x="APD 1 AO scale factor", y=w1521) -> (x*y=w1502:i16)
        n783 = Multiply(x="APD 2 AO scale factor", y=w1522) -> (x*y=w1501:i16)
        n784 = xnode "FPGA I/O Node"("Connector0/AO6"=w1502, "Connector0/AO7"=w1501) -> ()  [unwired: 2 in, 2 out]
      }
    }
  }
  n785 = disable-structure shown="Disabled" {
    disable-tunnel: w3 -> [w1540 _]
    frame Disabled {
      n786 = while "APD 3 Counter" {
        tunnel: w1540 -> [_]
        stop <- FALSE stop-if-true
        n787 = flat-sequence {
          frame #0 {
            n788 = xnode "FPGA I/O Method Node"("FPGA I/O In"=refnum<k21> "Connector0/DIO12" ("APD 2 DO"), "Timeout"=-1) -> ()  [unwired: 2 out]
          }
          frame #1 {
            n789 = local read "APD3 int gate"() -> (w1544:bool)
            n790 = case shown="True" w1544 {
              frame False {
              }
              frame True {
                n791 = local read item#-1() -> (w1545)
                n792 = case shown="True" w1545 {
                  frame False {
                    n793 = local read "APD 3 Counts 0"() -> (w1547:u32)
                    n794 = Increment(x=w1547) -> (x+1=→"APD 3 Counts 0":u32)
                  }
                  frame True {
                    n795 = local read "APD 3 Counts 1"() -> (w1549:u32)
                    n796 = Increment(x=w1549) -> (x+1=→"APD 3 Counts 1":u32)
                  }
                }
              }
            }
          }
        }
      }
    }
    frame Enabled {
    }
  }
  n797 = disable-structure shown="Disabled" {
    disable-tunnel: w3 -> [w1551 _]
    disable-tunnel: w5 -> [w1550 _]
    frame Disabled {
      n798 = while "APD 3 Gating" {
        shift-right: [w1555] -> _
        shift-left: w1551 -> [w1560]
        shift-right: [w1554] -> _
        shift-left: w1550 -> [w1552]
        stop <- FALSE stop-if-true
        n799 = flat-sequence {
          tunnel: w1560 -> [w1563]
          tunnel: [w1562] -> w1558
          tunnel: [w1563] -> w1556
          tunnel: [w1564] -> w1553
          tunnel: w1552 -> [w1564]
          tunnel: [w1567] -> w1559
          tunnel: w1558 -> [w1567]
          tunnel: [w1566] -> w1557
          tunnel: w1556 -> [w1566]
          tunnel: w1553 -> [w1565]
          tunnel: [w1588] -> w1555
          tunnel: w1559 -> [w1599]
          tunnel: w1557 -> [w1596]
          tunnel: [w1568] -> w1554
          frame #0 {
            n800 = call "Loop Timer5"("Count(Ticks)"=w1563) -> ("Tick Count(Ticks)"=w1562:u32)
          }
          frame #1 {
            # "Signal maybe then sent through \na transistor before APD"
            n801 = xnode "FPGA I/O Node"("Connector0/DIO2"=w1565) -> ()  [unwired: 1 in, 1 out]
            "APD3 int gate" <- w1565
          }
          frame #2 {
            n802 = local read "APD Gate OFF Count"() -> (w1573:u16)
            n803 = local read "APD Gate ON Count"() -> (w1574:u16)
            n804 = feedback #73(TRUE) -> (w1593:bool)
            n805 = feedback-in #74(w1599) -> ()
            n806 = feedback #74(w1599) -> (w1598:u32)
            n807 = Not(x=w1593) -> (.not. x?=w1591:bool)
            n808 = feedback-in #73(w1591) -> ()
            n809 = Subtract(x=w1599, y=w1598) -> (x-y=w1597:u32)
            n810 = Select(t=w1574, s=w1591, f=w1573) -> (s? t:f=w1595:u16)
            n811 = Subtract(x=w1597, y=w1596) -> (x-y=w1576:u32)
            n812 = Subtract(x=w1595, y=w1576) -> (x-y=w1587:u32)
            n813 = Number To Boolean Array(number=w1576) -> (Boolean array=w1577:bool[])
            n814 = Or Array Elements(Boolean array=w1577) -> (logical OR=w1575:bool)
            n815 = Boolean To (0,1)(Boolean=w1575) -> (0, 1=w1582:i16)
            n816 = Boolean To (0,1)(Boolean="+ phase (APD 3 Gate)") -> (0, 1=w1585:i16)
            n817 = To Unsigned Byte Integer(number=w1582) -> (unsigned 8bit integer=w1579:u8)
            n818 = Multiply(x=w1585, y="Phase count adjustment (APD 3 Gate)") -> (x*y=w1583:i16)
            n819 = feedback #75(u8 0) -> (w1580:u8)
            n820 = Add(x=w1579, y=w1580) -> (x+y=w1578:u8)
            "APD 3 Gate Late Counter" <- w1578
            n821 = feedback-in #75(w1578) -> ()
            n822 = Add(x=w1587, y=w1583) -> (x+y=w1588:u32)
            n823 = feedback #76(i16 0) -> (w1590:i16)
            n824 = Subtract(x=w1590, y=w1583) -> (x-y=w1589:i16)
            "APD 3 Gate Relative Phase" <- w1589
            n825 = feedback-in #76(w1589) -> ()
            n826 = local read "APD Gate Operating Mode"() -> (w1572:u8)
            n827 = case shown="2" w1572 {
              tunnel: [TRUE FALSE w1602] -> w1569
              tunnel: w1593 -> [_ _ w1602]
              frame 0, Default {
              }
              frame 1 {
              }
              frame 2 {
              }
            }
            n828 = local read "Invert APD Gate"() -> (w1571:bool)
            n829 = Not(x=w1569) -> (.not. x?=w1570:bool)
            n830 = Select(t=w1570, s=w1571, f=w1569) -> (s? t:f=w1568:bool)
          }
        }
      }
    }
    frame Enabled {
    }
  }
  n831 = disable-structure shown="Disabled" {
    disable-tunnel: w3 -> [w1605 _]
    disable-tunnel: w4 -> [w1604 _]
    frame Disabled {
      n832 = while "633 nm red  fluorescent laser interlacing (DO to IA 633 nm AOM ME amp)." {
        shift-right: [w1726] -> _
        shift-left: w1605 -> [w1731]
        shift-right: [w1725] -> _
        shift-left: w1604 -> [w1723]
        stop <- FALSE stop-if-true
        n833 = flat-sequence {
          tunnel: w1731 -> [w1734]
          tunnel: [w1733] -> w1729
          tunnel: [w1734] -> w1727
          tunnel: [w1735] -> w1724
          tunnel: w1723 -> [w1735]
          tunnel: [w1738] -> w1730
          tunnel: w1729 -> [w1738]
          tunnel: [w1737] -> w1728
          tunnel: w1727 -> [w1737]
          tunnel: w1724 -> [w1736]
          tunnel: [w1747] -> w1726
          tunnel: w1730 -> [w1767]
          tunnel: w1728 -> [w1764]
          tunnel: [w1756] -> w1725
          frame #0 {
            n834 = call "Loop Timer8"("Count(Ticks)"=w1734) -> ("Tick Count(Ticks)"=w1733:u32)
          }
          frame #1 {
            # "Then to PRL 440 amp"
            n835 = xnode "FPGA I/O Node"("Connector1/DIO32"=w1736) -> ()  [unwired: 1 in, 1 out]
          }
          frame #2 {
            n836 = feedback-in #77(w1767) -> ()
            n837 = feedback #77(w1767) -> (w1766:u32)
            n838 = Subtract(x=w1767, y=w1766) -> (x-y=w1765:u32)
            n839 = Subtract(x=w1765, y=w1764) -> (x-y=w1740:u32)
            n840 = Number To Boolean Array(number=w1740) -> (Boolean array=w1741:bool[])
            n841 = Or Array Elements(Boolean array=w1741) -> (logical OR=w1739:bool)
            n842 = Boolean To (0,1)(Boolean="+ phase (RI)") -> (0, 1=w1752:i16)
            n843 = Multiply(x=w1752, y="Phase count adjustment (RI)") -> (x*y=w1749:i16)
            n844 = Boolean To (0,1)(Boolean=w1739) -> (0, 1=w1746:i16)
            n845 = To Unsigned Byte Integer(number=w1746) -> (unsigned 8bit integer=w1743:u8)
            n846 = feedback #78(i16 0) -> (w1750:i16)
            n847 = feedback #79(u8 0) -> (w1744:u8)
            n848 = Add(x=w1743, y=w1744) -> (x+y=w1742:u8)
            "RI Late Counter" <- w1742
            n849 = feedback-in #79(w1742) -> ()
            n850 = Subtract(x=w1750, y=w1749) -> (x-y=w1748:i16)
            "RI Relative phase" <- w1748
            n851 = feedback-in #78(w1748) -> ()
            n852 = feedback #80(TRUE) -> (w1759:bool)
            n853 = case shown="2" "Red Laser Operating Mode" {
              tunnel: [TRUE FALSE w1773] -> w1756
              tunnel: w1759 -> [_ _ w1770]
              frame 0, Default {
              }
              frame 1 {
              }
              frame 2 {
                n854 = Not(x=w1770) -> (.not. x?=w1772:bool)
                n855 = Select(t=w1772, s="Invert RI", f=w1770) -> (s? t:f=w1773:bool)
              }
            }
            n856 = Not(x=w1759) -> (.not. x?=w1755:bool)
            n857 = Select(t="Red interlace ON count", s=w1755, f="Red interlace OFF count") -> (s? t:f=w1761:u16)
            n858 = Subtract(x=w1761, y=w1740) -> (x-y=w1753:u32)
            n859 = Add(x=w1753, y=w1749) -> (x+y=w1747:u32)
            n860 = feedback-in #80(w1755) -> ()
          }
        }
      }
      n861 = while "473 nm blue  fluorescent laser interlacing (DO to blue laser digital control input)." {
        shift-right: [w1622] -> _
        shift-left: w1605 -> [w1625]
        shift-right: [w1621] -> _
        shift-left: w1604 -> [w1619]
        shift-right: [w1614] -> _
        shift-left: _ -> [w1613]
        shift-right: [w1606] -> _
        shift-left: u16 0 -> [w1609]
        stop <- FALSE stop-if-true
        n862 = flat-sequence {
          tunnel: w1625 -> [w1628]
          tunnel: [w1627] -> w1624
          tunnel: [w1628] -> w1623
          tunnel: [w1631] -> w1620
          tunnel: w1619 -> [w1631]
          tunnel: w1613 -> [w1630]
          tunnel: [w1630] -> w1612
          tunnel: [w1629] -> w1610
          tunnel: w1609 -> [w1629]
          tunnel: [w1636] -> w1618
          tunnel: w1624 -> [w1636]
          tunnel: [w1635] -> w1617
          tunnel: w1623 -> [w1635]
          tunnel: w1620 -> [w1634]
          tunnel: w1612 -> [w1633]
          tunnel: [w1633] -> w1611
          tunnel: w1610 -> [w1632]
          tunnel: [w1632] -> w1608
          tunnel: [w1641] -> w1616
          tunnel: [w1640] -> w1615
          tunnel: w1617 -> [w1640]
          tunnel: w1618 -> [w1641]
          tunnel: w1611 -> [w1639]
          tunnel: w1608 -> [w1638]
          tunnel: [w1637] -> w1607
          tunnel: [w1698] -> w1622
          tunnel: w1616 -> [w1716]
          tunnel: w1615 -> [w1713]
          tunnel: [w1686] -> w1621
          tunnel: [w1684] -> w1614
          tunnel: w1607 -> [w1681]
          tunnel: [w1682] -> w1606
          frame #0 {
            n863 = call "Loop Timer7"("Count(Ticks)"=w1628) -> ("Tick Count(Ticks)"=w1627:u32)
          }
          frame #1 {
            n864 = xnode "FPGA I/O Node"("Connector1/DIO28"=w1634) -> ()  [unwired: 1 in, 1 out]
          }
          frame #2 {
            n865 = case shown="True" w1639 {
              tunnel: w1638 -> [w1642 w1644]
              tunnel: [w1642 w1643] -> w1637
              frame False {
              }
              frame True {
                n866 = flat-sequence {
                  tunnel: [w1650] -> w1647
                  tunnel: [w1649] -> w1646
                  tunnel: [w1648] -> w1645
                  tunnel: w1644 -> [w1648]
                  tunnel: w1647 -> [w1667]
                  tunnel: w1646 -> [w1664]
                  tunnel: w1645 -> [w1666]
                  tunnel: [w1665] -> w1643
                  frame #0 {
                    # "5 ns timing resolution"
                    n867 = node-c288() -> (w1653:T7)  [unwired: 1 in]
                    n868 = timed-loop {
                      timing: w1653 -> [_]
                      timing-out: [_] -> w1652
                      tunnel: "Lifetime timeout APD1" -> [w1659]
                      tunnel: [w1654] -> w1649
                      tunnel: [w1655] -> w1650
                      i -> [w1656]
                      stop <- w1658 stop-if-true
                      n869 = xnode "FPGA I/O Node"() -> ("Connector0/DIO5"=w1657:bool)  [unwired: 1 in, 1 out]
                      n870 = To Unsigned Word Integer(number=w1656) -> (unsigned 16bit integer=w1654:u16)
                      n871 = Equal?(x=w1659, y=w1654) -> (x = y?=w1655:bool)
                      n872 = Or(x=w1657, y=w1655) -> (x .or. y?=w1658:bool)
                    }
                    n873 = node-c288(w1652) -> ()
                  }
                  frame #1 {
                    n874 = Not(x=w1667) -> (.not. x?=w1668:bool)
                    n875 = case shown="True" w1668 {
                      tunnel: w1664 -> [_ w1670]
                      tunnel: w1666 -> [w1669 w1672]
                      tunnel: [w1669 w1671] -> w1665
                      frame False {
                        # "timed out, do nothing"
                      }
                      frame True {
                        # "photon detected,record time"
                        n876 = case shown="True" "Lifetime to FIFO" {
                          tunnel: w1670 -> [_ w1678]
                          tunnel: w1672 -> [w1674 w1676]
                          tunnel: [w1674 w1675] -> w1671
                          frame False {
                            # "don't record time\n(can't if doing force feedback)"
                          }
                          frame True {
                            # "number of events in fifo"
                            n877 = xnode ("FIFO Method Node")("Element"=w1678, "Timeout"=0) -> ()  [unwired: 1 in, 2 out]
                            n878 = Increment(x=w1676) -> (x+1=w1675:u16)
                          }
                        }
                        "lifetime (ticks)" <- w1670
                      }
                    }
                  }
                }
              }
            }
          }
          frame #3 {
            # "Reading fifo is tricky here since\nunknown # of events"
            # "For lifetime measurement:\nInterlacing and pulse falling"
            n879 = feedback-in #81(w1716) -> ()
            n880 = feedback #81(w1716) -> (w1715:u32)
            n881 = Subtract(x=w1716, y=w1715) -> (x-y=w1714:u32)
            n882 = Subtract(x=w1714, y=w1713) -> (x-y=w1691:u32)
            n883 = Number To Boolean Array(number=w1691) -> (Boolean array=w1692:bool[])
            n884 = Or Array Elements(Boolean array=w1692) -> (logical OR=w1690:bool)
            n885 = Boolean To (0,1)(Boolean="+ phase (BI D)") -> (0, 1=w1703:i16)
            n886 = Multiply(x=w1703, y="Phase count adjustment (BI D)") -> (x*y=w1700:i16)
            n887 = Boolean To (0,1)(Boolean=w1690) -> (0, 1=w1697:i16)
            n888 = To Unsigned Byte Integer(number=w1697) -> (unsigned 8bit integer=w1694:u8)
            n889 = feedback #82(i16 0) -> (w1701:i16)
            n890 = feedback #83(u8 0) -> (w1695:u8)
            n891 = Add(x=w1694, y=w1695) -> (x+y=w1693:u8)
            "Blue Late Counter (D)" <- w1693
            n892 = feedback-in #83(w1693) -> ()
            n893 = Subtract(x=w1701, y=w1700) -> (x-y=w1699:i16)
            "BI Relative phase (D)" <- w1699
            n894 = feedback-in #82(w1699) -> ()
            n895 = feedback #84(TRUE) -> (w1708:bool)
            n896 = case shown="2" "Blue Laser Operating Mode (D)" {
              tunnel: [TRUE FALSE w1722] -> w1686
              tunnel: w1708 -> [_ _ w1719]
              frame 0, Default {
              }
              frame 1 {
              }
              frame 2 {
                n897 = Not(x=w1719) -> (.not. x?=w1721:bool)
                n898 = Select(t=w1721, s="Invert BI (D)", f=w1719) -> (s? t:f=w1722:bool)
              }
            }
            n899 = Subtract(x=w1681, y="Lifetime events to read blue") -> (x-y=w1679:u16)
            n900 = Not(x=w1708) -> (.not. x?=w1706:bool)
            n901 = Select(t="Blue interlace ON count (D)", s=w1706, f="Blue interlace OFF count (D)") -> (s? t:f=w1710:u16)
            n902 = Subtract(x=w1710, y=w1691) -> (x-y=w1704:u32)
            n903 = Add(x=w1704, y=w1700) -> (x+y=w1698:u32)
            n904 = feedback-in #84(w1706) -> ()
            n905 = Select(t=w1679, s="Lifetime read blue fifo", f=w1681) -> (s? t:f=w1682:u16)
            "lifetime events in fifo" <- w1682
            n906 = Equal?(x="Blue Laser Operating Mode (D)", y=u8 2) -> (x = y?=w1687:bool)
            n907 = Not(x=w1686) -> (.not. x?=w1685:bool)
            n908 = And(x=w1685, y=w1687) -> (x .and. y?=w1684:bool)
          }
        }
      }
    }
    frame Enabled {
    }
  }
